vi "Amb_Factorial.vi"() -> ()   [LabVIEW 2015]
uses:
  <vilib>/Platform/TimedLoop/XDataNode/timing_clust.ctl
  <vilib>/Platform/TimedLoop/XDataNode/nitl_modes.ctl
  <vilib>/Platform/TimedLoop/XDataNode/wakeup.ctl
  <vilib>/DAQmx/read.llb/DAQmx Read (Analog DBL 1Chan 1Samp).vi
  <vilib>/DAQmx/read.llb/DAQmx Read (Analog 1D DBL NChan 1Samp).vi
  <vilib>/DAQmx/create/channels.llb/DAQmx Create Channel (AI-Voltage-Basic).vi
  <vilib>/Enthought/Python Integration Toolkit/api/Unpack Double.vi
  <vilib>/DAQmx/miscellaneous.llb/DAQmx Fill In Error Info.vi
  <vilib>/Platform/TimedLoop/XDataNode/XDataNode.xnode
  Program Files/neMESYS_SDK/neMESYS LabVIEW Kit/neMESYS LabVIEW Integration Kit.lvlib
  <vilib>/Platform/TimedLoop/XDataNode/XDNodeRunTimeDep.lvlib
  Conor/Temp CN7500/Omega CN7500/Omega CN7500.lvlib
  <vilib>/Enthought/Python Integration Toolkit/Python Integration Toolkit.lvlib
panel:
  out "Chi Sq 8":dbl
  out "Chi Sq ref 8":dbl
  out "Param 3 8":dbl
  out "Param 2 8":dbl
  out "Param 1 8":dbl
  out "Chi Sq 7":dbl
  out "Chi Sq ref 7":dbl
  out "Param 3 7":dbl
  out "Param 2 7":dbl
  out "Param 1 7":dbl
  out "Chi Sq 6":dbl
  out "Chi Sq ref 6":dbl
  out "Param 3 6":dbl
  out "Param 2 6":dbl
  out "Param 1 6":dbl
  out "Chi Sq 5":dbl
  out "Chi Sq ref 5":dbl
  out "Param 3 5":dbl
  out "Param 2 5":dbl
  out "Param 1 5":dbl
  out "Chi Sq 4":dbl
  out "Chi Sq ref 4":dbl
  out "Param 3 4":dbl
  out "Param 2 4":dbl
  out "Param 1 4":dbl
  in  "Cat Diameter um (eg 825)":dbl
  in  "Cat Mass G (EG 0.1)":dbl
  out "Exp 2":bool
  out "C EB 1":dbl
  out "C BAcid 1":dbl
  out "Exp 9":bool
  out "Liquid Inlet Pressure (bar g)":dbl
  in  "Liquid P sensor Terminal Configuration":i32(ring)=-1 items=["default"=-1, "RSE"=10083, "NRSE"=10078, "Differential"=10106, "Pseudodifferential"=12529]
  in  "Liquid P sensor Physical Channel":tag="Dev1/ai0"
  in  "Temp 2":dbl
  in  "Conc 2":dbl
  in  "Flow 2":dbl
  out "Exp 8":bool
  out "Exp 7":bool
  out "Exp 6":bool
  out "Exp 5":bool
  out "Exp 4":bool
  out "Exp 3":bool
  out "Exp 1":bool
  out "Exp 0":bool
  out "C BAcid 8":dbl
  out "C EB 8":dbl
  in  "Flow 8":dbl
  in  "Conc 8":dbl
  in  "Temp 8":dbl
  out "Temp 8":dbl
  out "Flow 8":dbl
  out "Conc 8":dbl
  out "C BAcid 7":dbl
  out "C EB 7":dbl
  in  "Flow 7":dbl
  in  "Conc 7":dbl
  in  "Temp 7":dbl
  out "Temp 7":dbl
  out "Flow 7":dbl
  out "Conc 7":dbl
  out "C BAcid 6":dbl
  out "C EB 6":dbl
  in  "Flow 6":dbl
  in  "Conc 6":dbl
  in  "Temp 6":dbl
  out "Temp 6":dbl
  out "Flow 6":dbl
  out "Conc 6":dbl
  out "C BAcid 5":dbl
  out "C EB 5":dbl
  in  "Flow 5":dbl
  in  "Conc 5":dbl
  in  "Temp 5":dbl
  out "Temp 5":dbl
  out "Flow 5":dbl
  out "Conc 5":dbl
  out "C BAcid 4":dbl
  out "C EB 4":dbl
  out "Conc 1":dbl
  out "Flow 1":dbl
  out "Temp 1":dbl
  out "Conc 2":dbl
  out "Flow 2":dbl
  out "Temp 2":dbl
  in  "Flow 4":dbl
  in  "Conc 4":dbl
  in  "Temp 4":dbl
  out "Temp 4":dbl
  out "Flow 4":dbl
  out "Conc 4":dbl
  out "C BAcid 3":dbl
  out "C EB 3":dbl
  out "Conc 3":dbl
  out "Flow 3":dbl
  out "Temp 3":dbl
  out "C BAcid 2":dbl
  out "C EB 2":dbl
  in  "Temp 3":dbl
  in  "Conc 3":dbl
  in  "Flow 3":dbl
  in  "Result file name -  needs extension .xlsx":string
  in  "HPLC file Name -doesnt need extension":string
  out "Desired Conc Not Possible":bool
  in  "Safety or Emergency Syringe Control":bool
  out "Feed Concentration (M)":dbl
  out "Total Flowrate (uL/min)":dbl
  out "Gas Back Pressure (barg)":dbl
  in  "Shut down in empty?\nLeft off, right on":bool
  in  "Clear":bool
  out "Safety Shut Down Pressure (barg)":dbl
  out "Calculated Pressure":dbl[](graph)
  out "Safety Shut Down Temp":dbl
  out "Actual Temp (oC)":dbl
  out "Temperature":dynamicdata(graph)
  out "Temp Set Point (oC)":dbl
  in  "Temp 1":dbl
  in  "Temp 0":dbl
  in  "Update Temperature Set Point":bool
  in  "Automated Experiments or Direct Control":bool
  in  "Set Point (oC)":dbl
  out "loop ind":dbl
  in  "Stop everything":bool
  in  "Skip Exp":bool
  in  "Minutes between Exp":dbl min=0.0 step=0.05
  in  "Refill 4":bool
  in  "Refill 3":bool
  in  "Refill 2":bool
  in  "Refill 1":bool
  in  "Empty 4":bool
  in  "Empty 3":bool
  in  "Empty 2":bool
  in  "Empty 1":bool
  in  "Calibrate 4":bool
  in  "Calibrate 3":bool
  in  "Calibrate 2":bool
  in  "Calibrate 1":bool
  in  "Stop Dose 4":bool
  in  "Stop Dose 3":bool
  in  "Stop Dose 2":bool
  in  "Stop Dose 1":bool
  in  "Flow 1":dbl
  in  "Conc 1":dbl
  in  "Flow 0":dbl
  in  "Conc 0":dbl
  in  "Generate Flow":bool
  in  "Set Flowrate 1":dbl
  in  "Set Flowrate 2":dbl
  in  "Set Flowrate 3":dbl
  in  "Set Flowrate 4":dbl
  in  "High Conc":dbl min=0.0 max=2.0
  in  "Low Conc":dbl min=0.0 max=2.0
  out "Syringe Level 4":dbl(slide) scale=0.0..5500.0
  out "Syringe Level 3":dbl(slide) scale=0.0..5500.0
  out "Syringe Level 2":dbl(slide) scale=0.0..5500.0
  out "Syringe Level 1":dbl(slide) scale=0.0..5500.0
  out "Flowrate 4 High":dbl
  out "Flowrate 3 High":dbl
  out "Flowrate 2 Low":dbl
  out "Flowrate 1 Low":dbl
  # "Pre Planned Experiments"
  # "Conducted Experiments Set Points"
  # "Current Conditions"
  # "1 & 2 chosen in advance"
  # "(uL/min)"
  # "3 onwards MBDoE"
  # "Coerced to nearest possible"
  # "Reported Values are set point no actual\nso if set point is not possible\ncoercion takes place\nbut actual is not recorded"
  # "Experimental Info"
  # "Factorial Only"
  # "example file name to show correct format is..."
  # "MBDoE2peakin1"
  # "Direct Control"
  # "Emergency Syringe Control Below"
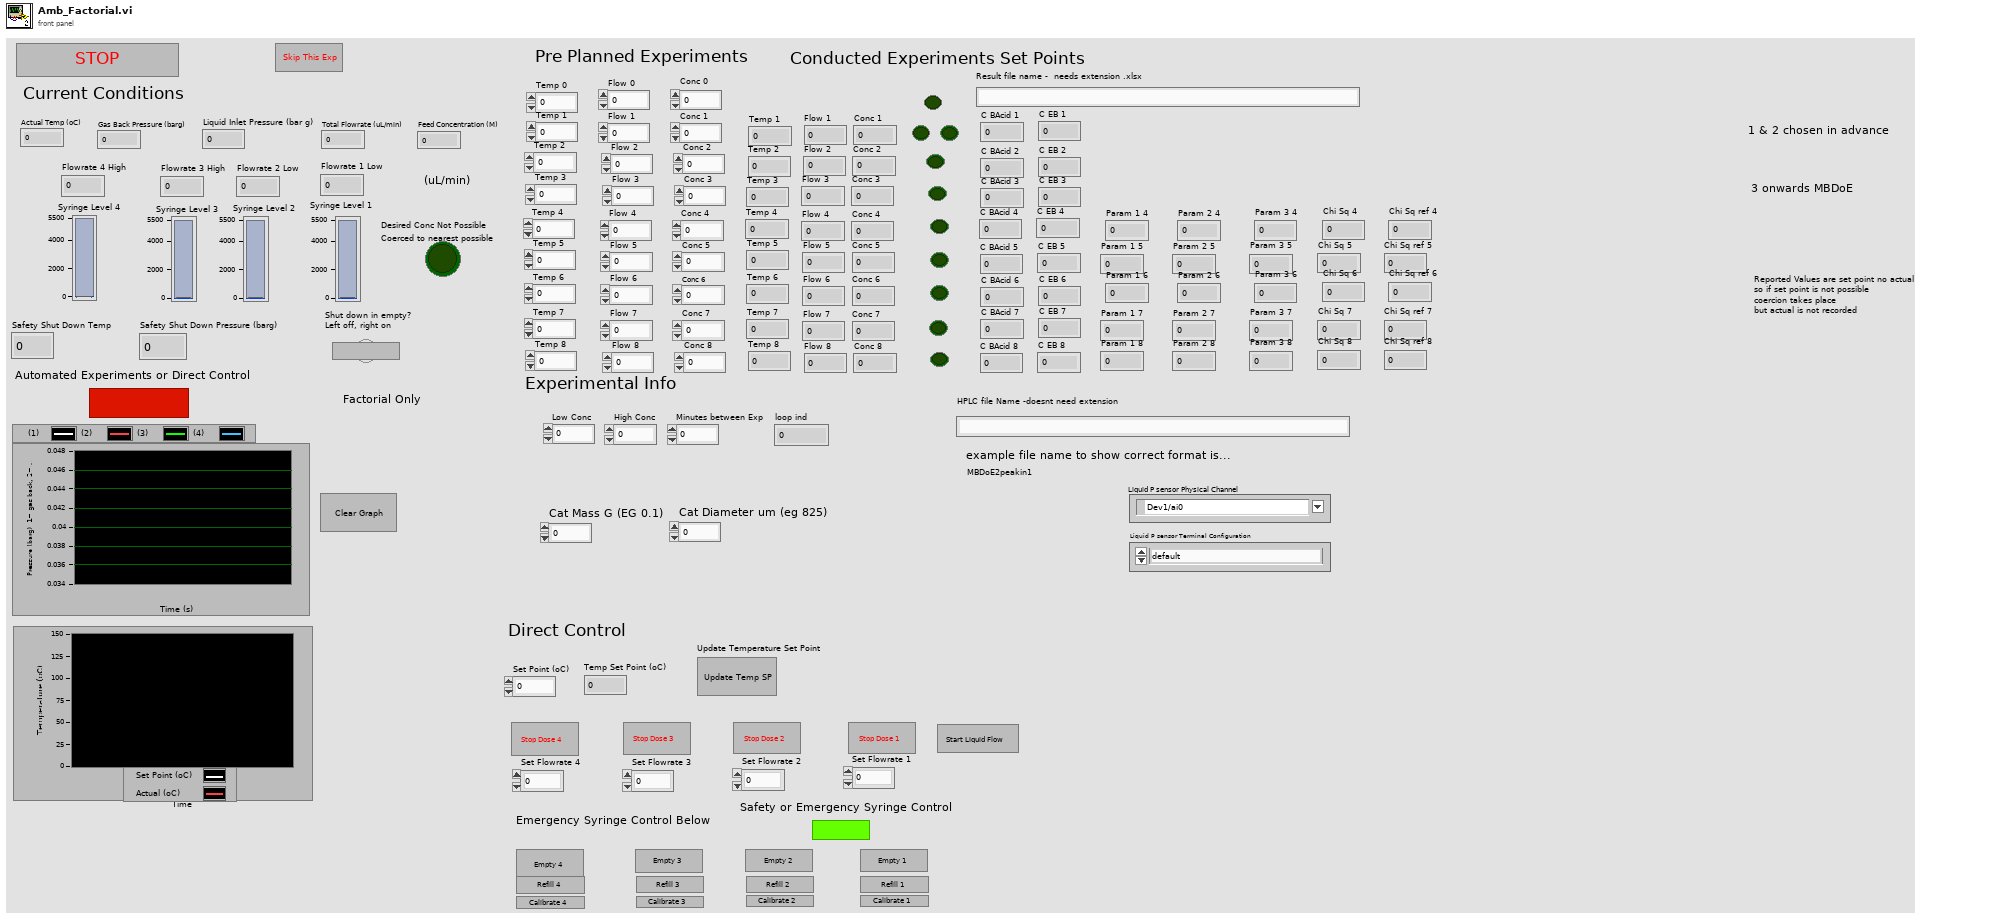
[diagram p1: front panel]
types:
  T1 = typedef "XDNodeRunTimeDep.lvlib/timing_clust.ctl" = cluster{"Expected End [f-1]":u64, "Actual End [f-1]":u64, "Finished Late? [f-1]":bool, "Expected End [i-1]":u64, "Actual End [i-1]":u64, "Finished Late? [i-1]":bool, "Expected Start [i]":u64, "Actual Start [i]":u64, "Expected Start [f]":u64, "Actual Start [f]":u64, "Source Name":string, "Structure Name":string, "Period":i64, "Deadline":i64, "Offset":i64, "Start":i64, "Priority":i32, "Timeout":i32, "Mode":T2, "Wakeup Reason":T3, "Error":errorcluster, "Source Type":string, "Secondary Source Type":string, "Global End Time":u64, "Global Start Time":u64, "Frame Duration":u64, "Iteration Duration":u64, "Assigned CPU":i32, "I/O Scan Engine Mode":u32}
  T2 = typedef "XDNodeRunTimeDep.lvlib/nitl_modes.ctl" = enum32{"No Change", "Process missed periods, maintain original phase", "Discard missed periods, maintain original phase", "Process missed periods, ignore original phase", "Discard missed periods, ignore original phase"}
  T3 = typedef "XDNodeRunTimeDep.lvlib/wakeup.ctl" = enum32{"Normal", "Aborted", "Asynchronous wakeup", "Timing source error", "Timed loop error", "Timeout"}
  T4 = typedef "Python Integration Toolkit.lvlib/Session ID.ctl" = u64
  T5 = typedef "Python Integration Toolkit.lvlib/Python Objects.ctl" = variant
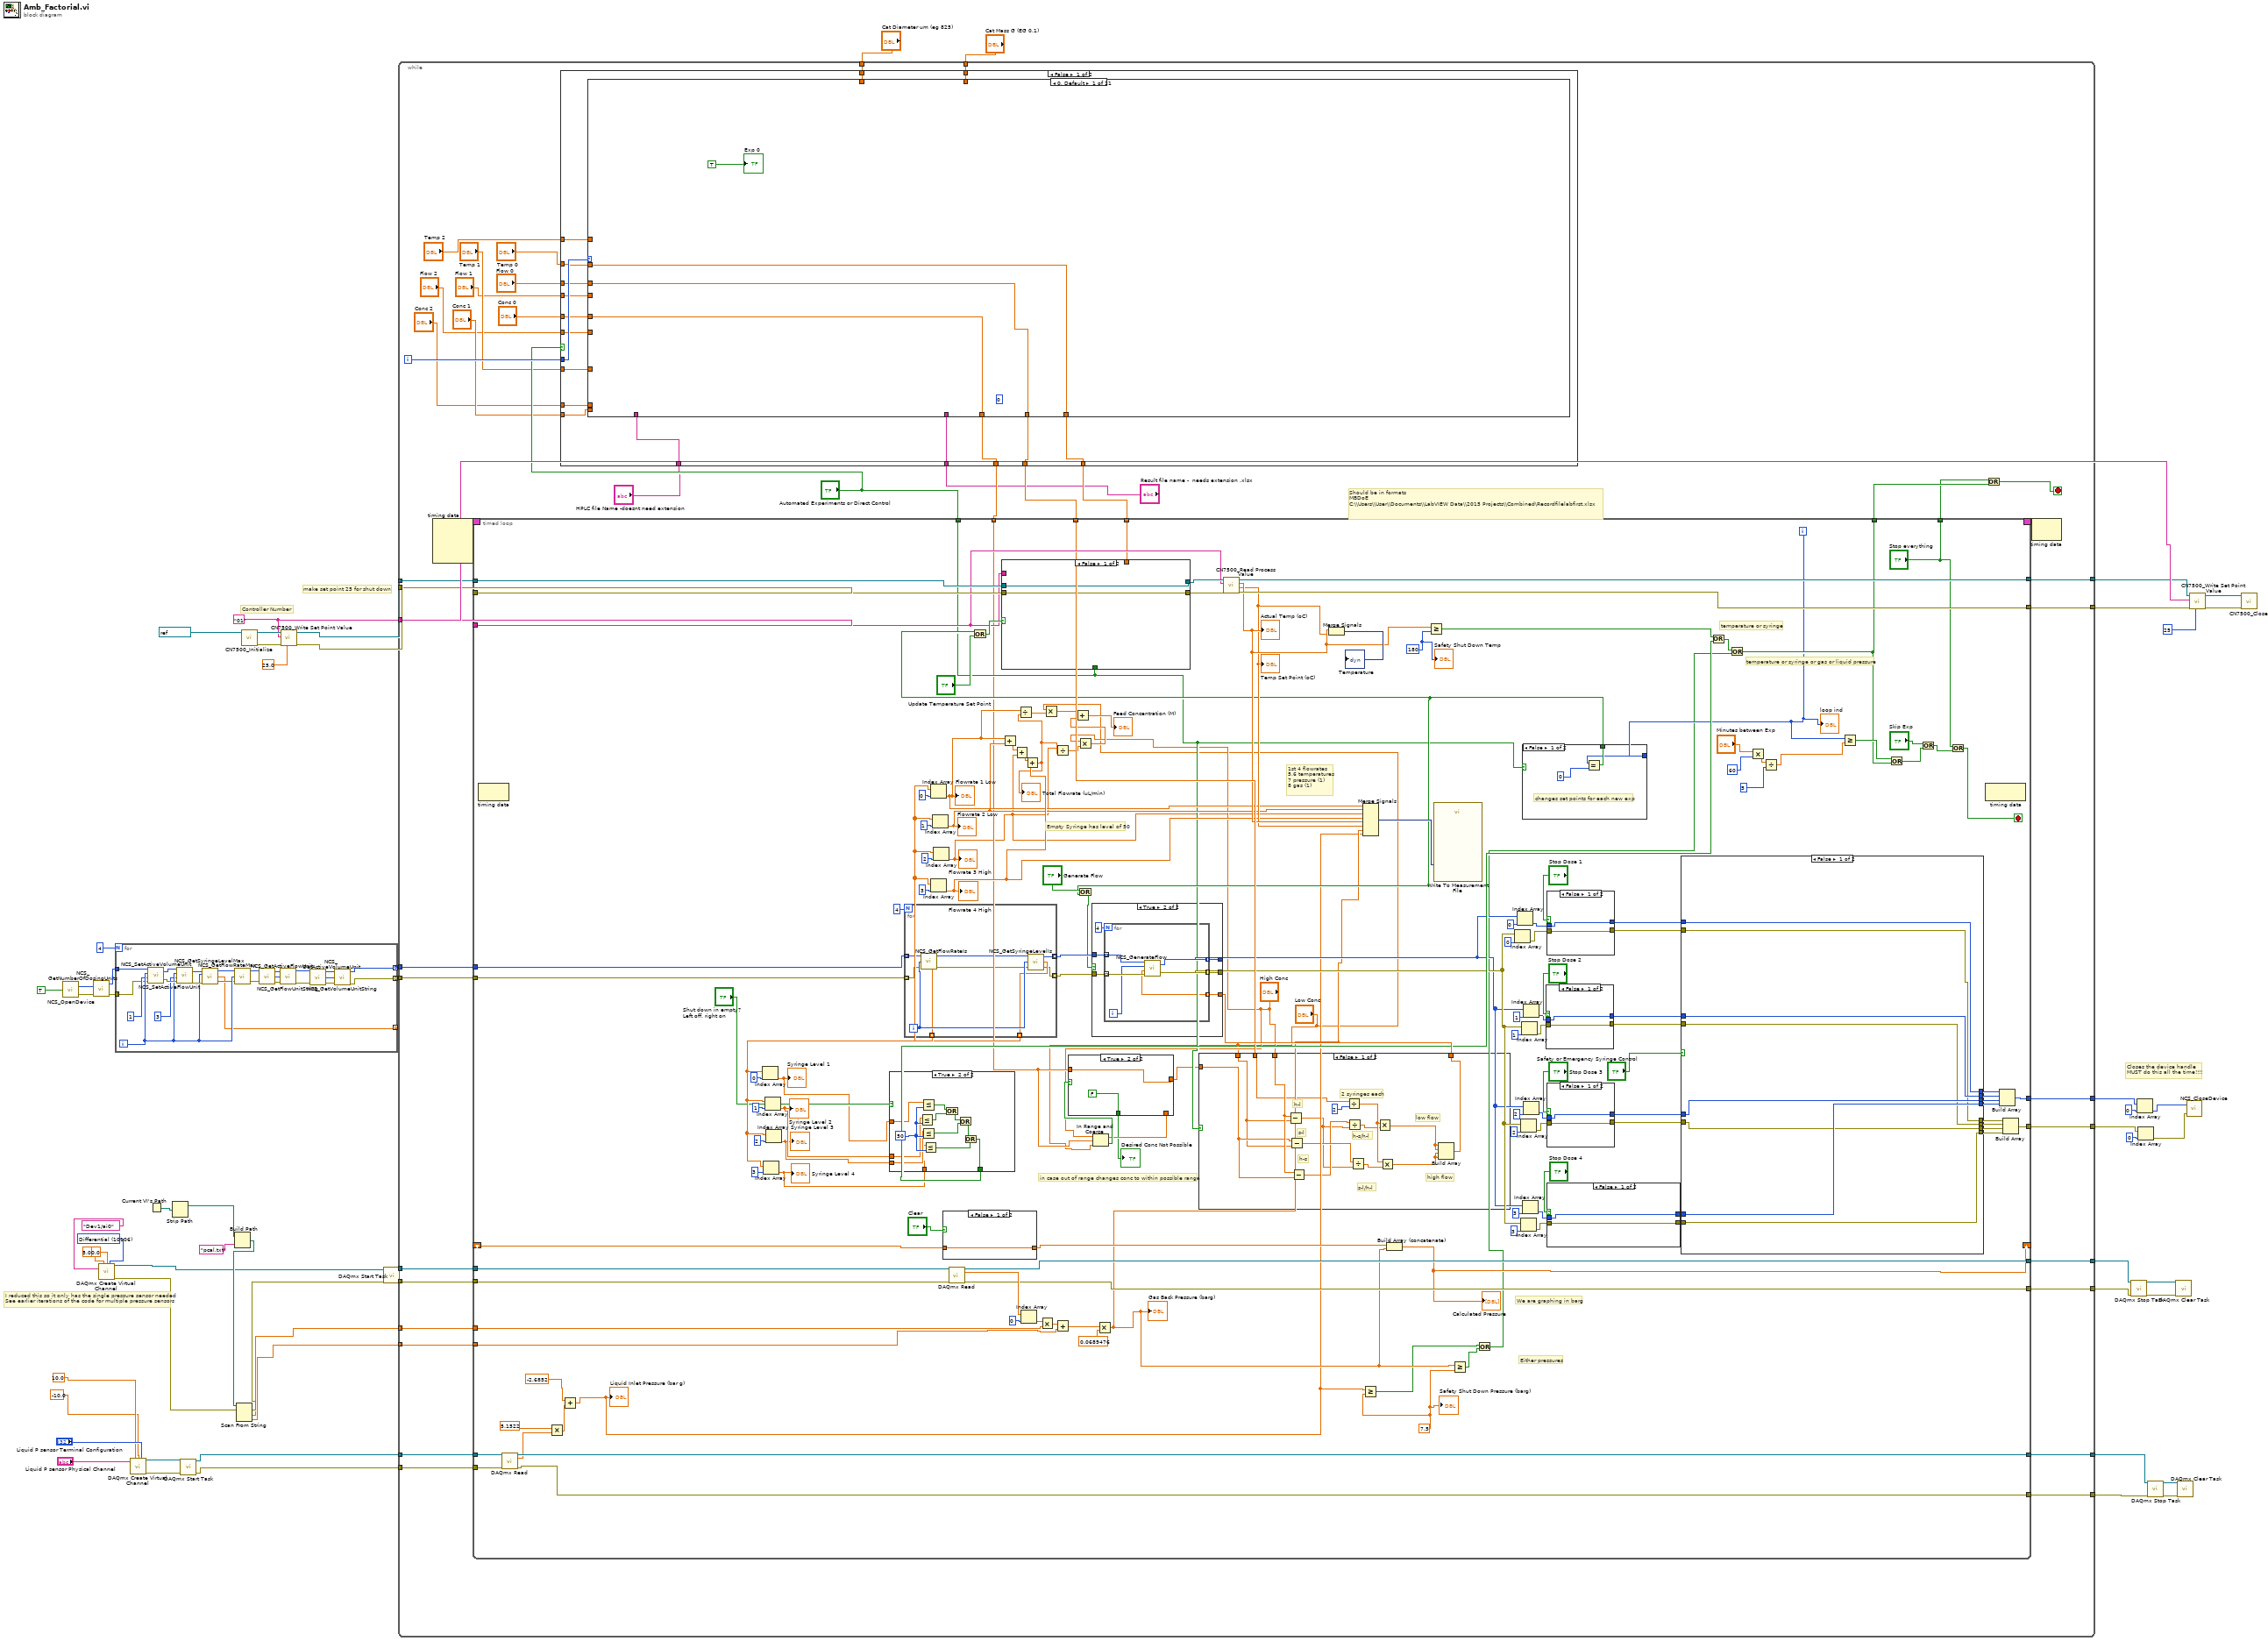
[diagram p0: block diagram]
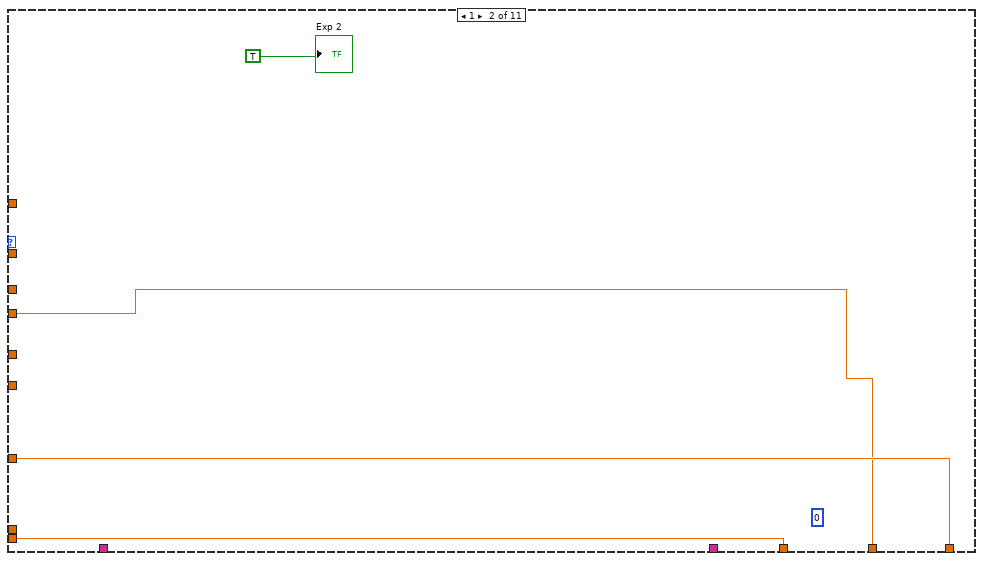
[diagram p2: hidden frame]
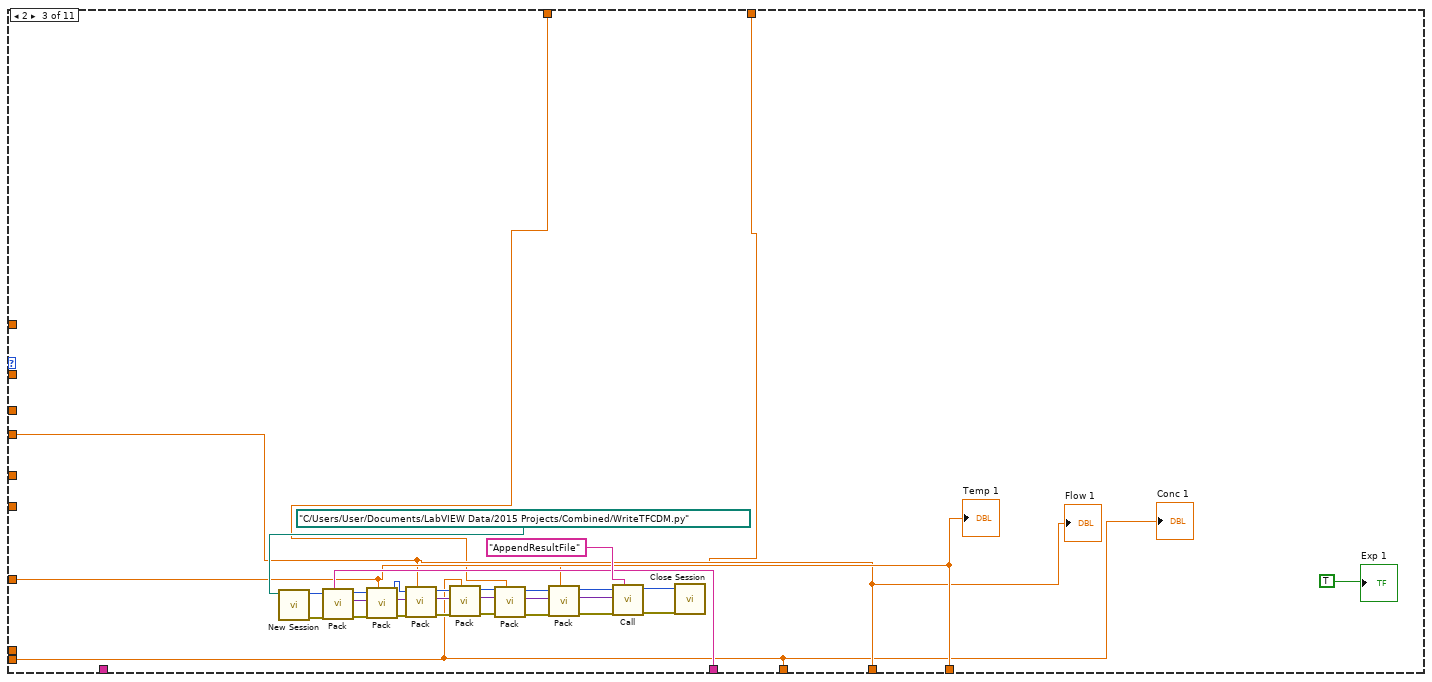
[diagram p3: hidden frame]
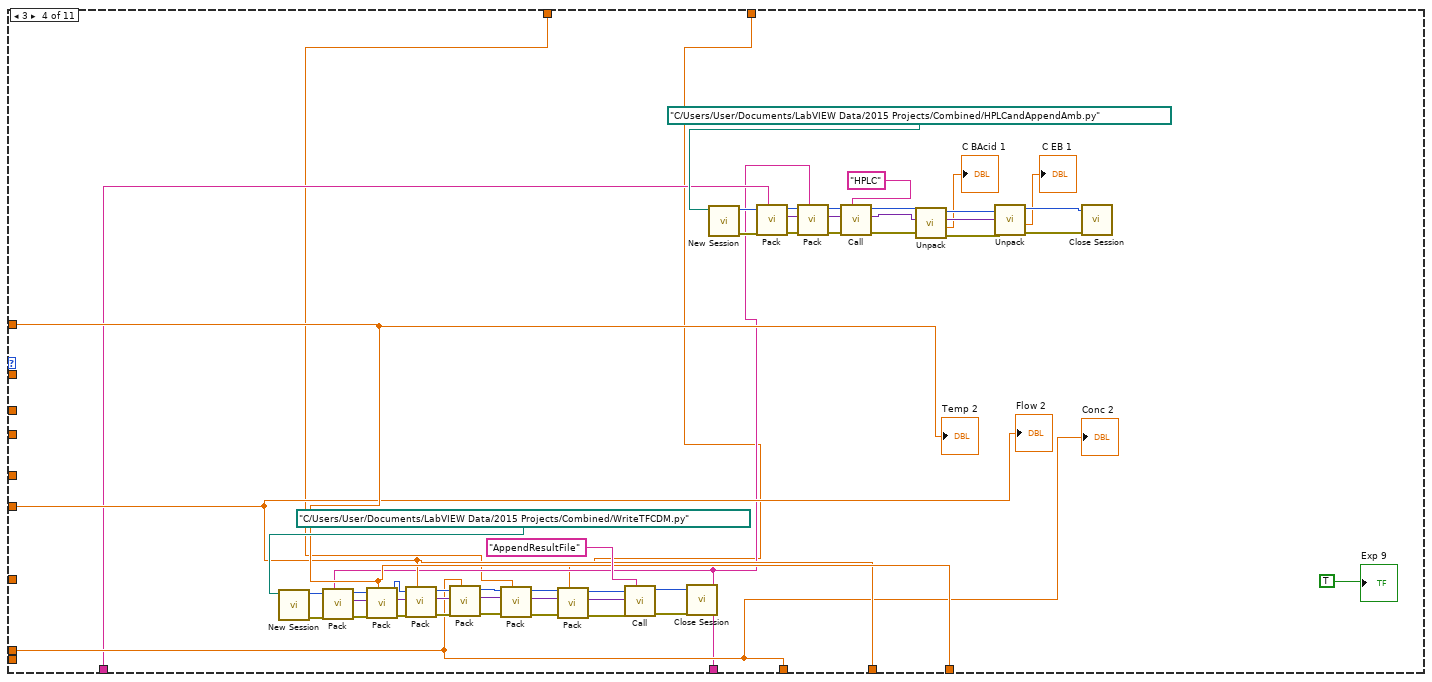
[diagram p4: hidden frame]
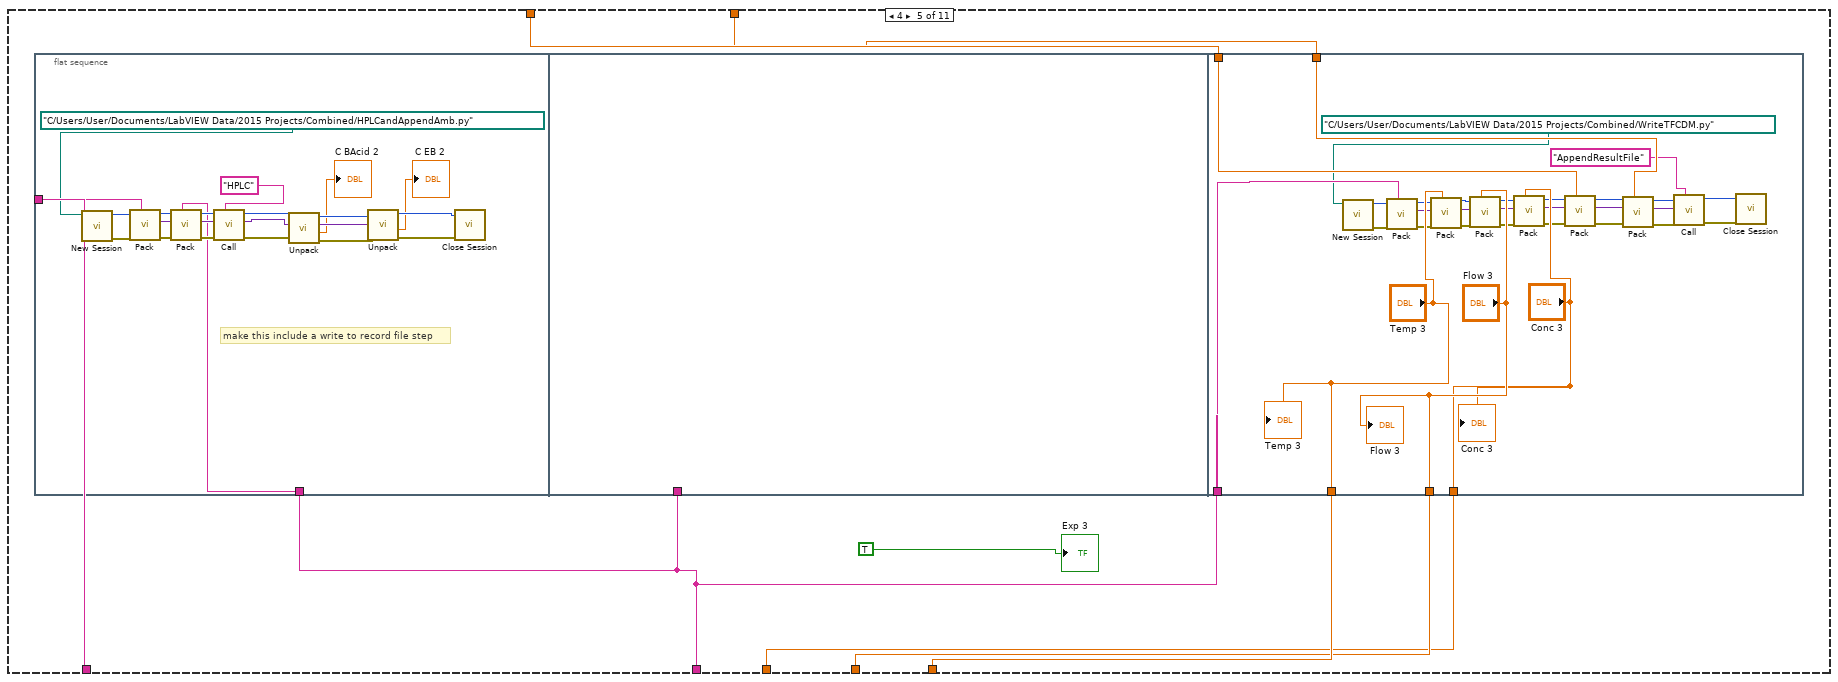
[diagram p5: hidden frame]
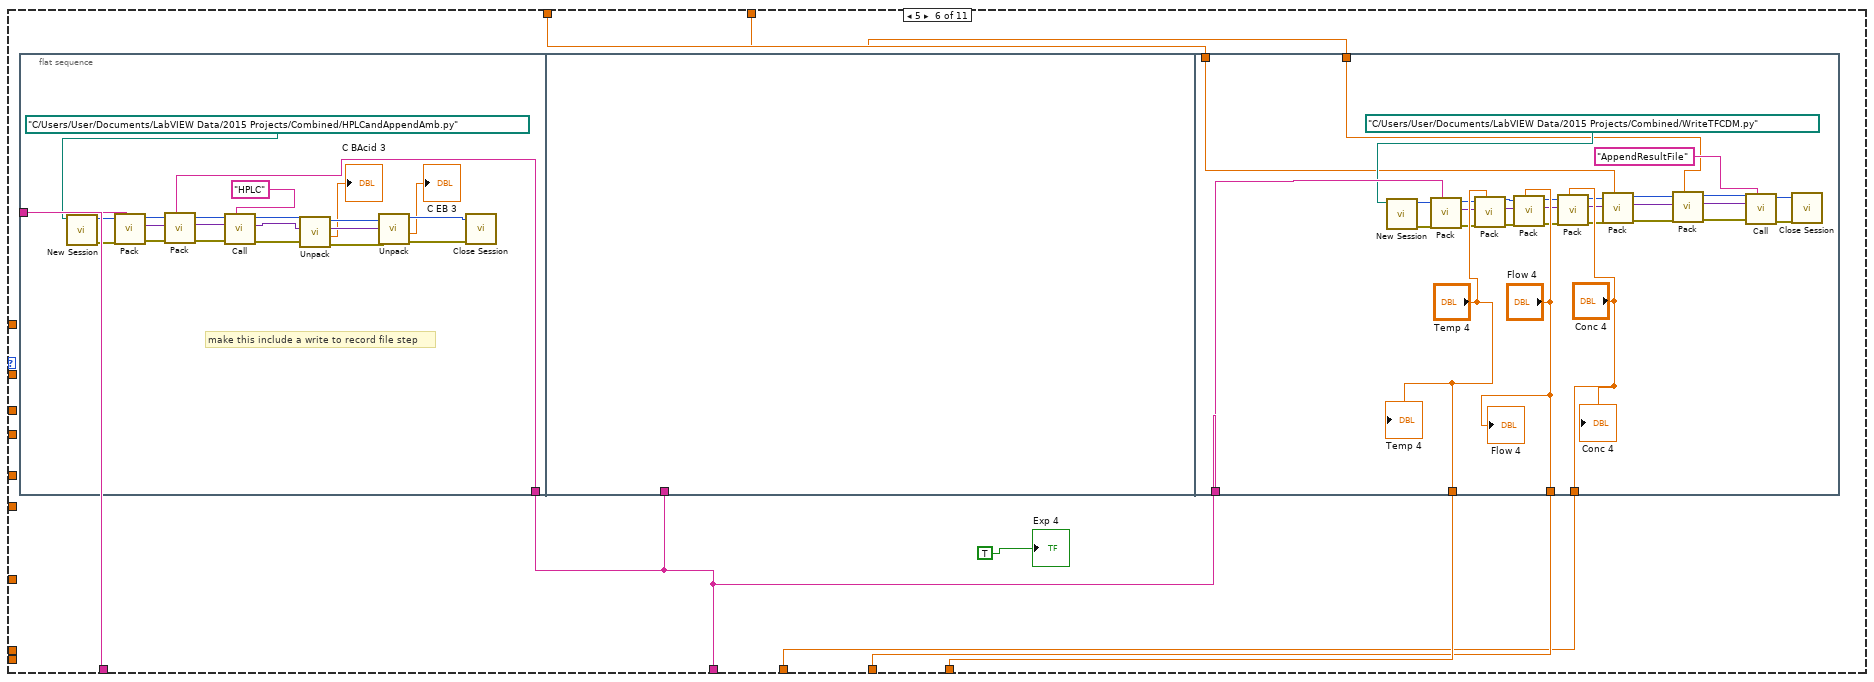
[diagram p6: hidden frame]
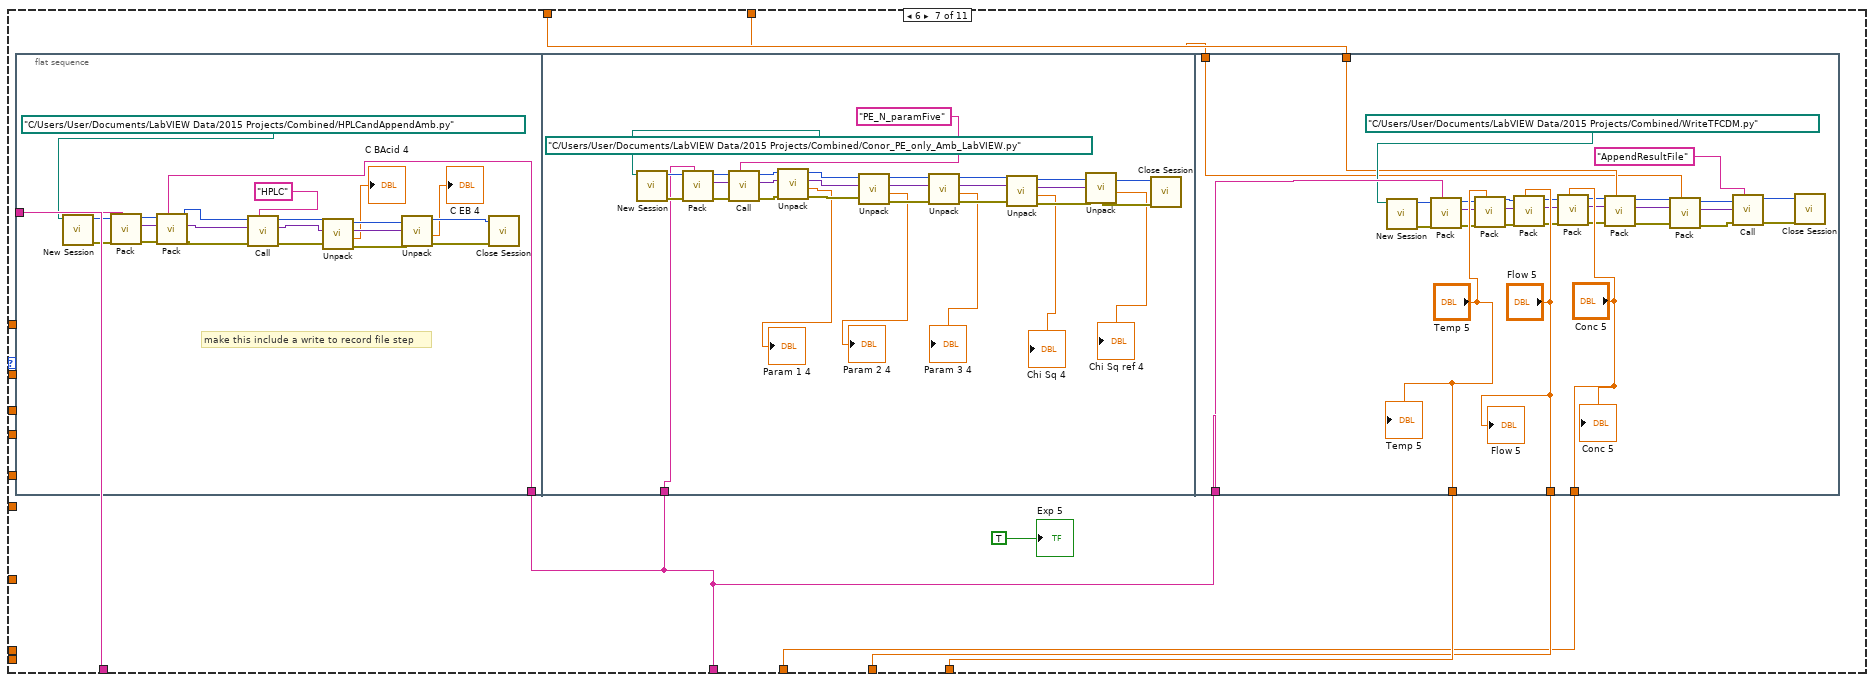
[diagram p7: hidden frame]
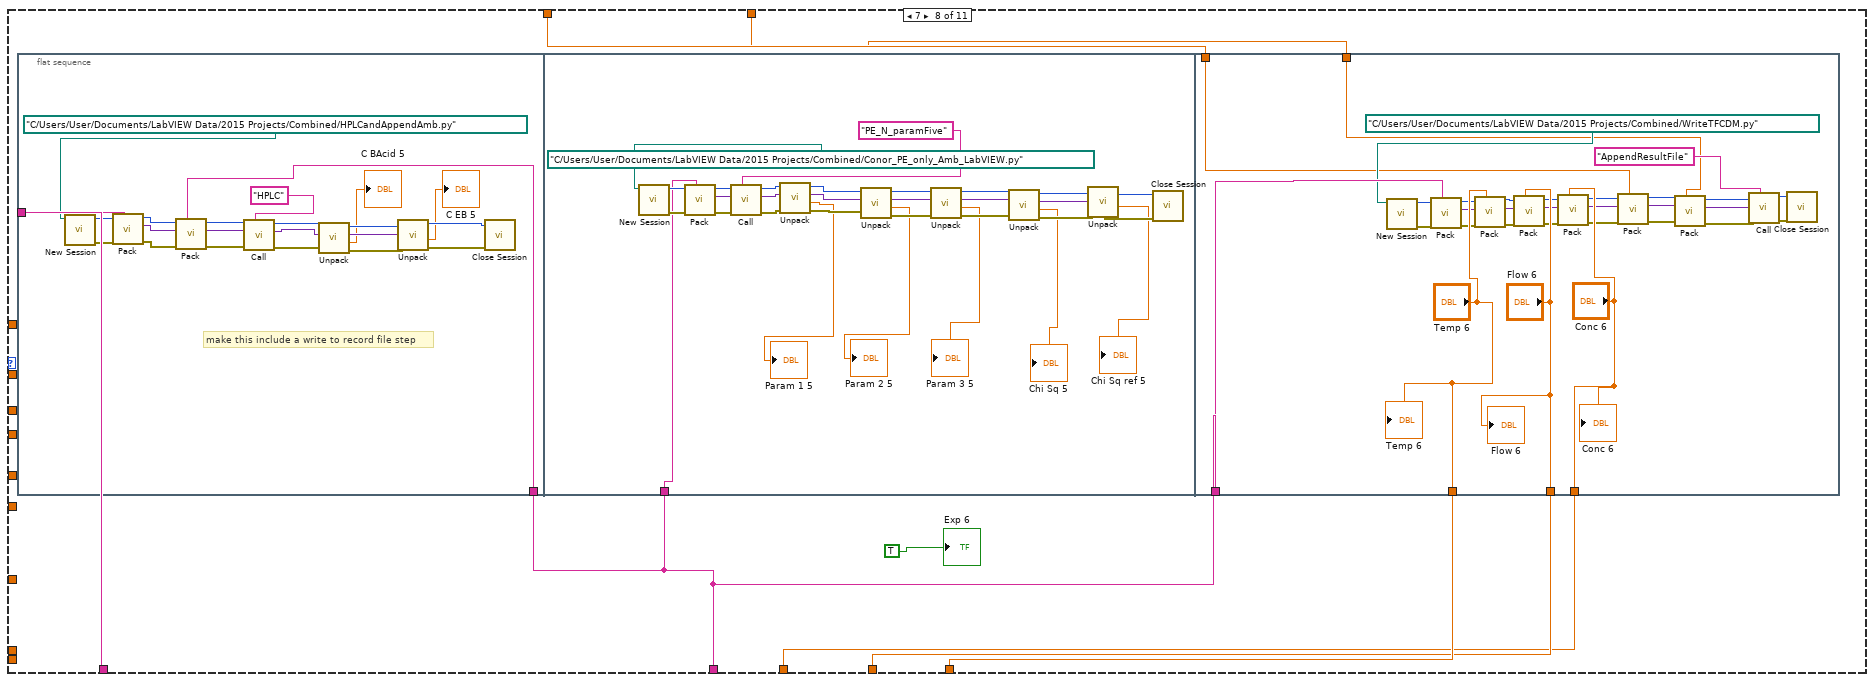
[diagram p8: hidden frame]
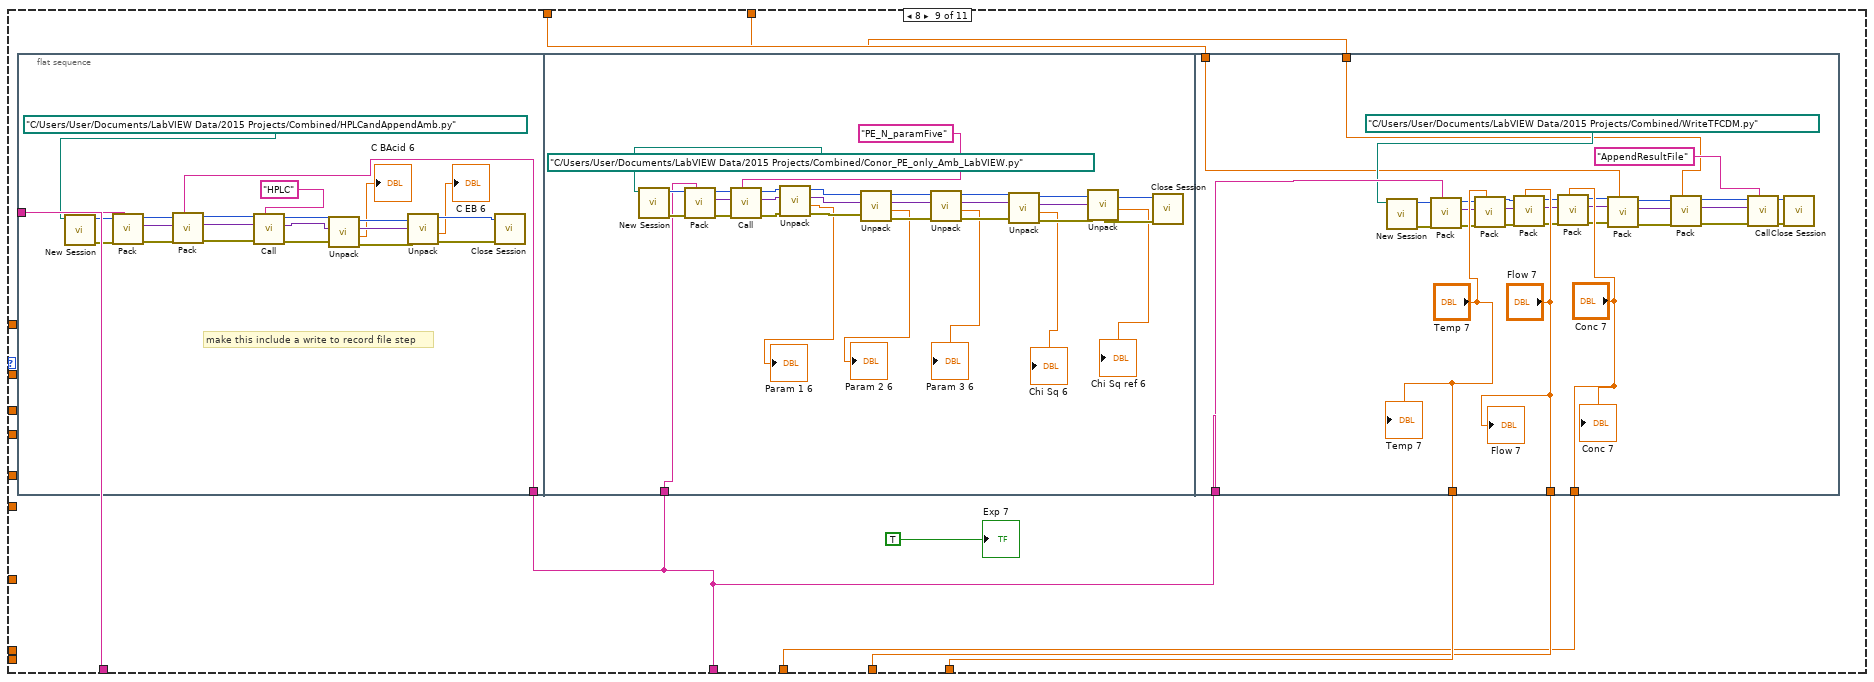
[diagram p9: hidden frame]
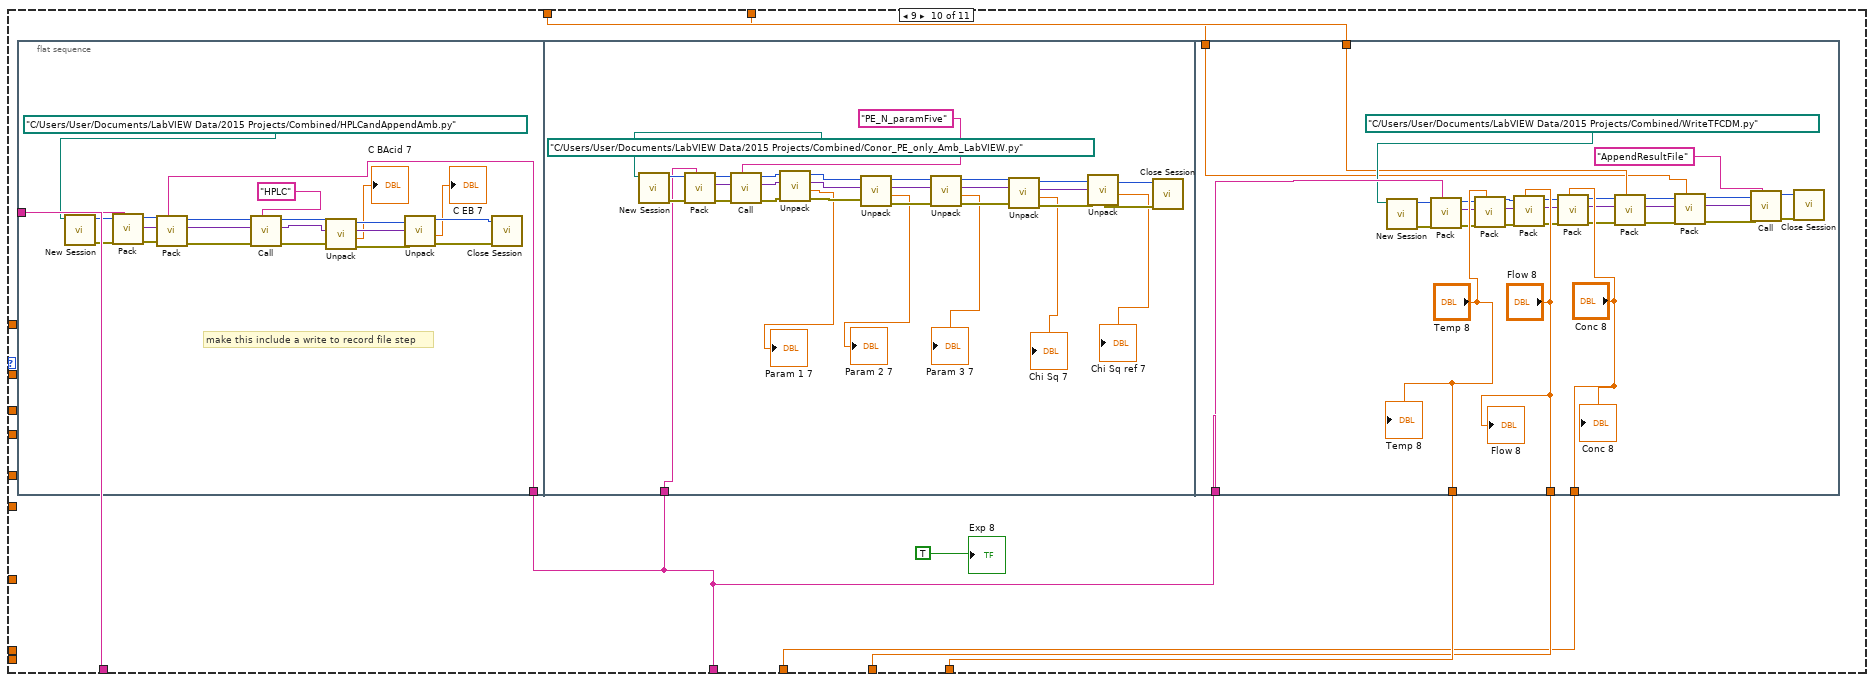
[diagram p10: hidden frame]
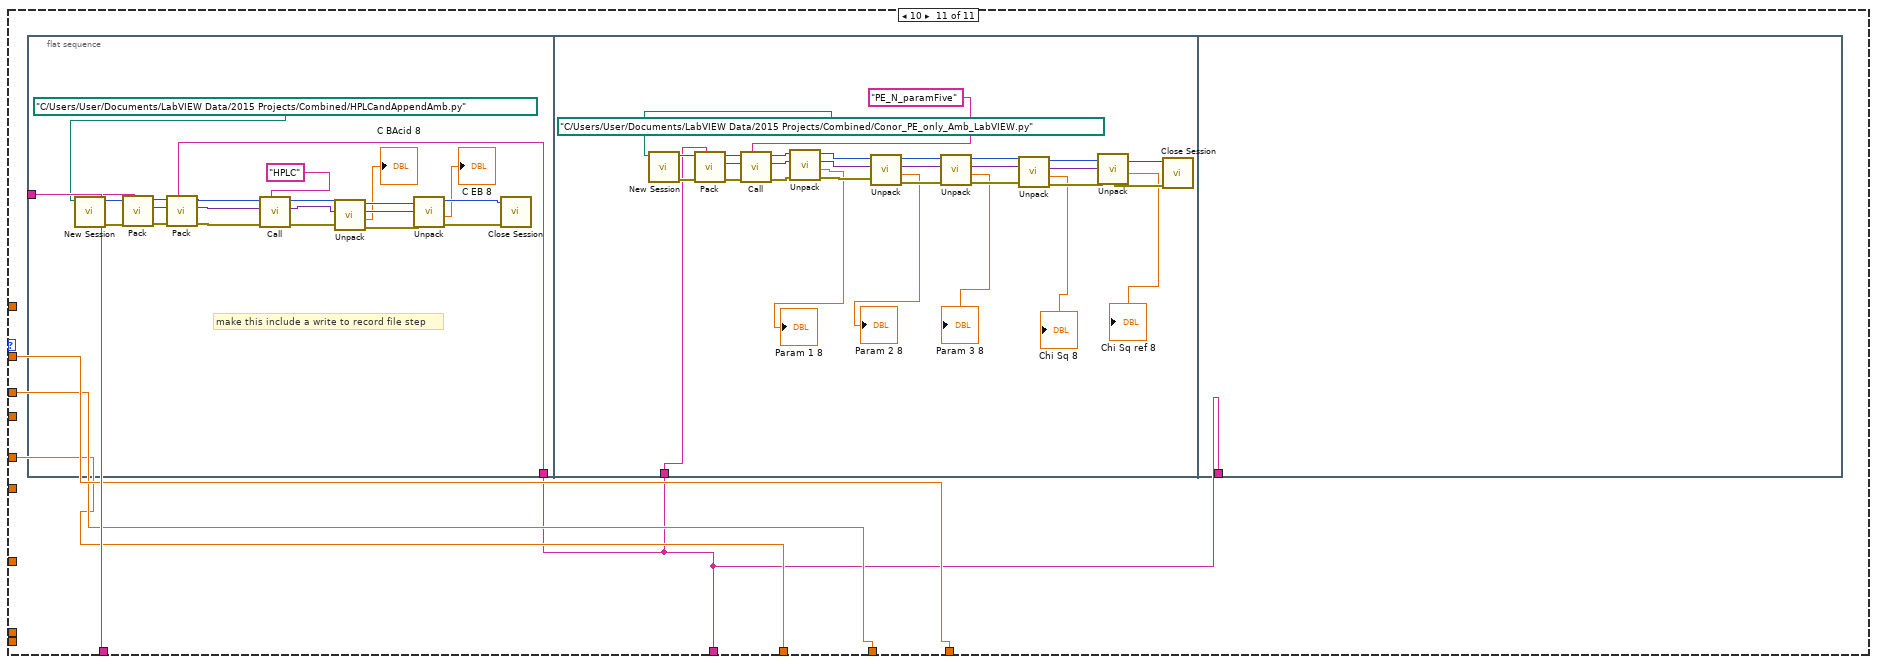
[diagram p11: hidden frame]
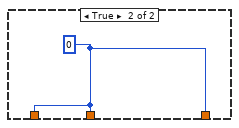
[diagram p12: hidden frame]
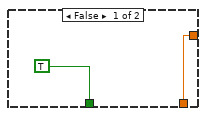
[diagram p13: hidden frame]
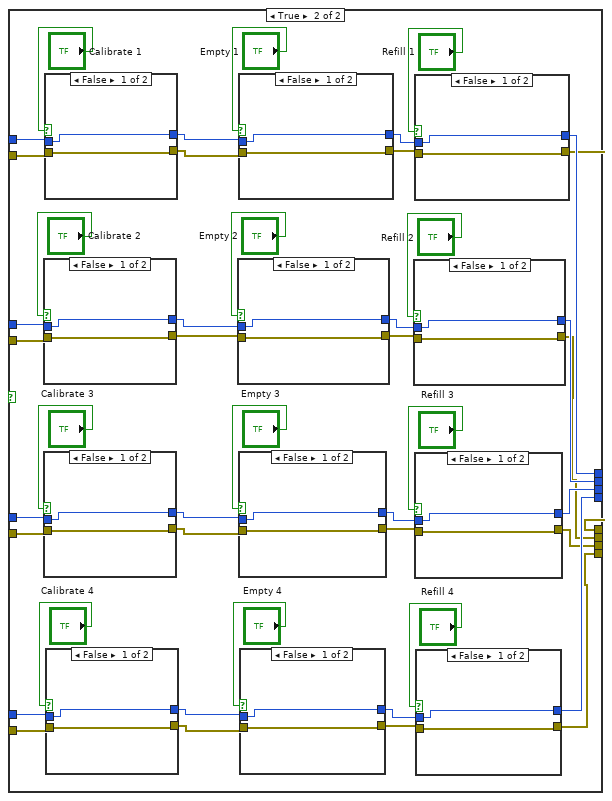
[diagram p14: hidden frame]
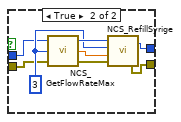
[diagram p15: hidden frame]
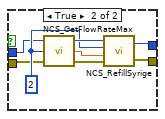
[diagram p16: hidden frame]
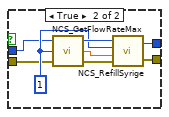
[diagram p17: hidden frame]
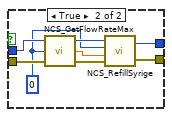
[diagram p18: hidden frame]
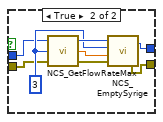
[diagram p19: hidden frame]
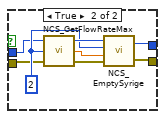
[diagram p20: hidden frame]
diagram:
  w31 = 10106 items=["default"=-1, "RSE"=10083, "NRSE"=10078, "Differential"=10106, "Pseudodifferential"=12529] ("input terminal configuration")
  w38 = "01" ("Controller Number")
  # "I reduced this so it only has the single pressure sensor needed\nSee earlier iterations of the code for multiple pressure sensors"
  # "make set point 25 for shut down"
  # "Controller Number"
  # "Closes the device handle \nMUST do this all the time!!!!"
  n1 = call "NCS_OpenDevice.vi"("show status window"=TRUE) -> ("device handle"=w57:u32, "error out"=w56:errorcluster)
  n2 = call "NCS_GetNumberOfDosingUnits.vi"("device handle in"=w57, "error in (no error)"=w56) -> ("device handle out"=w54:u32, "error out"=w55:errorcluster)  [unwired: 1 out]
  n3 = call-poly <vilib>:"DAQmx Create Virtual Channel.vi"("maximum value"=5.0, "minimum value"=0.0, "input terminal configuration"=w31, "physical channels"=tag "Dev1/ai0") -> ("task out"=w15:refnum<k21>, "error out"=w16:errorcluster)  [unwired: 10 in]
  n4 = for {
    N: 4 -> [_]
    tunnel: [w63] -> w53 mode=indexing
    tunnel: [w62] -> w52 mode=indexing
    tunnel: [w76] -> _ mode=indexing
    tunnel: w55 -> [w61]
    tunnel: w54 -> [w60]
    i -> [w79]
    n5 = call "NCS_SetActiveVolumeUnit.vi"("error in (no error)"=w61, "active volume unit"=1, "dosingunit"=w79, "device handle in"=w60) -> ("error out"=w82:errorcluster, "device handle out"=w83:u32)
    n6 = call "NCS_SetActiveFlowUnit.vi"("error in (no error)"=w82, "active flow unit"=3, "dosingunit"=w79, "device handle in"=w83) -> ("error out"=w80:errorcluster, "device handle out"=w81:u32)
    n7 = call "NCS_GetSyringeLevelMax.vi"("error in (no error)"=w80, "dosingunit"=w79, "device handle in"=w81) -> ("error out"=w77:errorcluster, "syringe level max"=w76:dbl, "device handle out"=w78:u32)  [unwired: 1 out]
    n8 = call "NCS_GetFlowRateMax.vi"("error in (no error)"=w77, "dosingunit"=w79, "device handle in"=w78) -> ("error out"=w64:errorcluster, "device handle out"=w65:u32)  [unwired: 1 out]
    n9 = call "NCS_GetActiveFlowUnit.vi"("error in (no error)"=w64, "device handle in"=w65) -> ("error out"=w72:errorcluster, "active flow unit"=w71:u8, "device handle out"=w73:u32)  [unwired: 1 in]
    n10 = call "NCS_GetFlowUnitString.vi"("device handle in"=w73, "flow unit id"=w71, "error in (no error)"=w72) -> ("device handle out"=w68:u32, "error out"=w67:errorcluster)  [unwired: 2 out]
    n11 = call "NCS_GetActiveVolumeUnit.vi"("error in (no error)"=w67, "device handle in"=w68) -> ("error out"=w69:errorcluster, "active volume unit"=w70:u8, "device handle out"=w66:u32)  [unwired: 1 in]
    n12 = call "NCS_GetVolumeUnitString.vi"("device handle in"=w66, "volume unit id"=w70, "error in (no error)"=w69) -> ("device handle out"=w63:u32, "error out"=w62:errorcluster)  [unwired: 2 out]
  }
  n13 = call-poly <vilib>:"DAQmx Create Virtual Channel.vi"("maximum value"=10.0, "minimum value"=-10.0 ("maximum value"), "input terminal configuration"="Liquid P sensor Terminal Configuration", "physical channels"="Liquid P sensor Physical Channel") -> ("task out"=w11:refnum<k21>, "error out"=w12:errorcluster)  [unwired: 10 in]
  n14 = Current VI's Path() -> (path=w29:path)
  n15 = Strip Path(path=w29) -> (stripped path=w27:path)  [unwired: 1 out]
  n16 = call <vilib>:"DAQmx Start Task.vi"("task/channels in"=w11, "error in"=w12) -> ("task out"=w10:refnum<k21>, "error out"=w9:errorcluster)  [unwired: 12 in]
  n17 = Build Path(base path=w27, name or relative path="pcal.txt") -> (appended path=w28:path)
  n18 = Scan From String(w28, w16) -> (w25:errorcluster, output 1=w22:dbl, output 2=w21:dbl)  [unwired: 3 in, 1 out]
  n19 = call "CN7500_Initialize.vi"("VISA resource name"=refnum<visa-resource-name> "COM8") -> ("error out"=w44:errorcluster, "VISA resource name out"=w45:refnum<visa-resource-name>)  [unwired: 9 in]
  n20 = call "CN7500_Write Set Point Value.vi"("Target Set Point Value"=25.0, "error in (no error)"=w44, "Controller Number"=w38, "VISA In"=w45) -> ("error out"=w36:errorcluster, "VISA Out"=w37:refnum<visa-resource-name>)  [unwired: 6 in]
  n21 = call <vilib>:"DAQmx Start Task.vi"("task/channels in"=w15, "error in"=w25) -> ("task out"=w24:refnum<k21>, "error out"=w23:errorcluster)  [unwired: 12 in]
  n22 = while {
    tunnel: w53 -> [w125]
    tunnel: w52 -> [w124]
    tunnel: [w123] -> w47
    tunnel: [w122] -> w46
    tunnel: w38 -> [w119]
    tunnel: w37 -> [w118]
    tunnel: w36 -> [w117]
    tunnel: [w116] -> w35
    tunnel: [w115] -> w34
    tunnel: w24 -> [w113]
    tunnel: w23 -> [w112]
    tunnel: w22 -> [w111]
    tunnel: w21 -> [w110]
    tunnel: [w109] -> w18
    tunnel: [w108] -> w17
    tunnel: w10 -> [w92]
    tunnel: w9 -> [w91]
    tunnel: [w90] -> w7
    tunnel: [w89] -> w5
    tunnel: "Cat Diameter um (eg 825)" -> [w85]
    tunnel: "Cat Mass G (EG 0.1)" -> [w84]
    i -> [w102]
    stop <- w107 stop-if-true
    # "Should be in formats \nMBDoE\nC:\\\\Users\\\\User\\\\Documents\\\\LabVIEW Data\\\\2015 Projects\\\\Combined\\Recordfilelabfirst.xlsx"
    n23 = node-c288() -> (w121:T1)  [unwired: 4 in]
    n24 = case shown="False" "Automated Experiments or Direct Control" {
      tunnel: [w139 w771] -> w105
      tunnel: [w137 w771] -> w104
      tunnel: [w141 w771] -> w103
      tunnel: w102 -> [w142 _]
      tunnel: "Conc 0" -> [w140 _]
      tunnel: "Flow 0" -> [w136 _]
      tunnel: "Temp 0" -> [w138 _]
      tunnel: "Temp 1" -> [w134 _]
      tunnel: "Flow 1" -> [w133 _]
      tunnel: "Conc 1" -> [w132 _]
      tunnel: "HPLC file Name -doesnt need extension" -> [w131 _]
      tunnel: "Result file name -  needs extension .xlsx" -> [w135 _]
      tunnel: "Temp 2" -> [w130 _]
      tunnel: "Flow 2" -> [w129 _]
      tunnel: "Conc 2" -> [w128 _]
      tunnel: w85 -> [w127 _]
      tunnel: w84 -> [w126 _]
      frame False {
        n25 = case shown="0, Default" w142 {
          tunnel: [w144 w147 w163 w215 w238 w298 w358 w448 w538 w628 w715] -> w141
          tunnel: w140 -> [w144 _ _ _ _ _ _ _ _ _ w715]
          tunnel: [w146 w149 w165 w217 w240 w300 w360 w450 w540 w630 w717] -> w139
          tunnel: w138 -> [w146 _ _ _ _ _ _ _ _ _ w717]
          tunnel: [w145 w148 w164 w216 w239 w299 w359 w449 w539 w629 w716] -> w137
          tunnel: w136 -> [w145 _ _ _ _ _ _ _ _ _ w716]
          tunnel: w135 -> [_ _ w166 w193 w237 w297 w357 w447 w537 w627 w714]
          tunnel: w134 -> [_ w149 w165 _ _ _ _ _ _ _ _]
          tunnel: w133 -> [_ w148 w164 _ _ _ _ _ _ _ _]
          tunnel: w132 -> [_ w147 w163 _ _ _ _ _ _ _ _]
          tunnel: w131 -> [_ _ _ w194 w241 w301 w361 w451 w541 w631 w718]
          tunnel: w130 -> [_ _ _ w217 _ _ _ _ _ _ _]
          tunnel: w129 -> [_ _ _ w216 _ _ _ _ _ _ _]
          tunnel: w128 -> [_ _ _ w215 _ _ _ _ _ _ _]
          tunnel: w127 -> [_ _ w161 w183 w235 w295 w355 w445 w535 w625 _]
          tunnel: w126 -> [_ _ w160 w182 w234 w294 w354 w444 w534 w624 _]
          frame 0, Default {
            (unwired) 0
            "Exp 0" <- TRUE
          }
          frame 1 {
            (unwired) 0
            "Exp 2" <- TRUE
          }
          frame 2 {
            n26 = call <vilib>:"New Session.vi"("Path to Python Module (.py File)"=path "C:/Users/User/Documents/LabVIEW Data/2015 Projects/Combined/WriteTFCDM.py") -> ("error out"=w173:errorcluster, "Session ID out"=w172:T4)  [unwired: 9 in]
            n27 = call <vilib>:"Pack.vi"("Argument"=w166, "error in (no error)"=w173, "Session ID"=w172) -> ("error out"=w174:errorcluster, "Python Object References Out"=w178:T5, "Session ID out"=w171:T4)  [unwired: 6 in]
            n28 = call <vilib>:"Pack.vi"("Argument"=w165, "error in (no error)"=w174, "Python Object References In"=w178, "Session ID"=w171) -> ("error out"=w175:errorcluster, "Python Object References Out"=w179:T5, "Session ID out"=w181:T4)  [unwired: 5 in]
            n29 = call <vilib>:"Pack.vi"("Argument"=w164, "error in (no error)"=w175, "Python Object References In"=w179, "Session ID"=w181) -> ("error out"=w176:errorcluster, "Python Object References Out"=w180:T5, "Session ID out"=w167:T4)  [unwired: 5 in]
            n30 = call <vilib>:"Pack.vi"("Argument"=w163, "error in (no error)"=w176, "Python Object References In"=w180, "Session ID"=w167) -> ("error out"=w153:errorcluster, "Python Object References Out"=w156:T5, "Session ID out"=w159:T4)  [unwired: 5 in]
            n31 = call <vilib>:"Pack.vi"("Argument"=w161, "error in (no error)"=w153, "Python Object References In"=w156, "Session ID"=w159) -> ("error out"=w152:errorcluster, "Python Object References Out"=w155:T5, "Session ID out"=w158:T4)  [unwired: 5 in]
            n32 = call <vilib>:"Pack.vi"("Argument"=w160, "error in (no error)"=w152, "Python Object References In"=w155, "Session ID"=w158) -> ("error out"=w151:errorcluster, "Python Object References Out"=w154:T5, "Session ID out"=w157:T4)  [unwired: 5 in]
            n33 = call <vilib>:"Call.vi"("Function or Method Name"="AppendResultFile", "error in (no error)"=w151, "Python Object References In"=w154, "Session ID"=w157) -> ("error out"=w177:errorcluster, "Session ID out"=w168:T4)  [unwired: 5 in, 1 out]
            n34 = call <vilib>:"Close Session.vi"("error in (no error)"=w177, "Session ID"=w168) -> ()  [unwired: 9 in, 1 out]
            "Temp 1" <- w165
            "Flow 1" <- w164
            "Conc 1" <- w163
            "Exp 1" <- TRUE
          }
          frame 3 {
            n35 = call <vilib>:"New Session.vi"("Path to Python Module (.py File)"=path "C:/Users/User/Documents/LabVIEW Data/2015 Projects/Combined/WriteTFCDM.py") -> ("error out"=w225:errorcluster, "Session ID out"=w224:T4)  [unwired: 9 in]
            n36 = call <vilib>:"Pack.vi"("Argument"=w193, "error in (no error)"=w225, "Session ID"=w224) -> ("error out"=w226:errorcluster, "Python Object References Out"=w230:T5, "Session ID out"=w223:T4)  [unwired: 6 in]
            n37 = call <vilib>:"Pack.vi"("Argument"=w217, "error in (no error)"=w226, "Python Object References In"=w230, "Session ID"=w223) -> ("error out"=w227:errorcluster, "Python Object References Out"=w231:T5, "Session ID out"=w233:T4)  [unwired: 5 in]
            n38 = call <vilib>:"Pack.vi"("Argument"=w216, "error in (no error)"=w227, "Python Object References In"=w231, "Session ID"=w233) -> ("error out"=w228:errorcluster, "Python Object References Out"=w232:T5, "Session ID out"=w219:T4)  [unwired: 5 in]
            n39 = call <vilib>:"Pack.vi"("Argument"=w215, "error in (no error)"=w228, "Python Object References In"=w232, "Session ID"=w219) -> ("error out"=w186:errorcluster, "Python Object References Out"=w189:T5, "Session ID out"=w192:T4)  [unwired: 5 in]
            n40 = call <vilib>:"Pack.vi"("Argument"=w183, "error in (no error)"=w186, "Python Object References In"=w189, "Session ID"=w192) -> ("error out"=w185:errorcluster, "Python Object References Out"=w188:T5, "Session ID out"=w191:T4)  [unwired: 5 in]
            n41 = call <vilib>:"Pack.vi"("Argument"=w182, "error in (no error)"=w185, "Python Object References In"=w188, "Session ID"=w191) -> ("error out"=w184:errorcluster, "Python Object References Out"=w187:T5, "Session ID out"=w190:T4)  [unwired: 5 in]
            n42 = call <vilib>:"Call.vi"("Function or Method Name"="AppendResultFile", "error in (no error)"=w184, "Python Object References In"=w187, "Session ID"=w190) -> ("error out"=w229:errorcluster, "Session ID out"=w220:T4)  [unwired: 5 in, 1 out]
            n43 = call <vilib>:"Close Session.vi"("error in (no error)"=w229, "Session ID"=w220) -> ()  [unwired: 9 in, 1 out]
            n44 = call <vilib>:"New Session.vi"("Path to Python Module (.py File)"=path "C:/Users/User/Documents/LabVIEW Data/2015 Projects/Combined/HPLCandAppendAmb.py") -> ("error out"=w211:errorcluster, "Session ID out"=w210:T4)  [unwired: 9 in]
            n45 = call <vilib>:"Pack.vi"("Argument"=w194, "error in (no error)"=w211, "Session ID"=w210) -> ("error out"=w196:errorcluster, "Python Object References Out"=w198:T5, "Session ID out"=w200:T4)  [unwired: 6 in]
            n46 = call <vilib>:"Pack.vi"("Argument"=w193, "error in (no error)"=w196, "Python Object References In"=w198, "Session ID"=w200) -> ("error out"=w195:errorcluster, "Python Object References Out"=w197:T5, "Session ID out"=w199:T4)  [unwired: 5 in]
            n47 = call <vilib>:"Call.vi"("Function or Method Name"="HPLC", "error in (no error)"=w195, "Python Object References In"=w197, "Session ID"=w199) -> ("error out"=w212:errorcluster, "Python Object References Out"=w203:T5, "Session ID out"=w204:T4)  [unwired: 5 in]
            n48 = call-poly <vilib>:"Unpack.vi"("error in (no error)"=w212, "Python Object References In"=w203, "Session ID"=w204) -> ("error out"=w213:errorcluster, "Value"=→"C BAcid 1":dbl, "Python Object References Out"=w208:T5, "Session ID out"=w207:T4)  [unwired: 5 in]
            n49 = call-poly <vilib>:"Unpack.vi"("error in (no error)"=w213, "Python Object References In"=w208, "Session ID"=w207) -> ("error out"=w214:errorcluster, "Value"=→"C EB 1":dbl, "Session ID out"=w209:T4)  [unwired: 5 in, 1 out]
            n50 = call <vilib>:"Close Session.vi"("error in (no error)"=w214, "Session ID"=w209) -> ()  [unwired: 9 in, 1 out]
            "Exp 9" <- TRUE
            "Temp 2" <- w217
            "Flow 2" <- w216
            "Conc 2" <- w215
          }
          frame 4 {
            n51 = flat-sequence {
              tunnel: w241 -> [w249]
              tunnel: w237 -> [w242]
              tunnel: w237 -> [_]
              tunnel: w237 -> [w293]
              tunnel: ["Temp 3"] -> w240
              tunnel: ["Flow 3"] -> w239
              tunnel: ["Conc 3"] -> w238
              tunnel: w235 -> [w289]
              tunnel: w234 -> [w288]
              frame #0 {
                # "make this include a write to record file step"
                n52 = call <vilib>:"New Session.vi"("Path to Python Module (.py File)"=path "C:/Users/User/Documents/LabVIEW Data/2015 Projects/Combined/HPLCandAppendAmb.py") -> ("error out"=w260:errorcluster, "Session ID out"=w259:T4)  [unwired: 9 in]
                n53 = call <vilib>:"Pack.vi"("Argument"=w249, "error in (no error)"=w260, "Session ID"=w259) -> ("error out"=w244:errorcluster, "Python Object References Out"=w246:T5, "Session ID out"=w248:T4)  [unwired: 6 in]
                n54 = call <vilib>:"Pack.vi"("Argument"=w242, "error in (no error)"=w244, "Python Object References In"=w246, "Session ID"=w248) -> ("error out"=w243:errorcluster, "Python Object References Out"=w245:T5, "Session ID out"=w247:T4)  [unwired: 5 in]
                n55 = call <vilib>:"Call.vi"("Function or Method Name"="HPLC", "error in (no error)"=w243, "Python Object References In"=w245, "Session ID"=w247) -> ("error out"=w261:errorcluster, "Python Object References Out"=w252:T5, "Session ID out"=w253:T4)  [unwired: 5 in]
                n56 = call-poly <vilib>:"Unpack.vi"("error in (no error)"=w261, "Python Object References In"=w252, "Session ID"=w253) -> ("error out"=w262:errorcluster, "Value"=→"C BAcid 2":dbl, "Python Object References Out"=w257:T5, "Session ID out"=w256:T4)  [unwired: 5 in]
                n57 = call-poly <vilib>:"Unpack.vi"("error in (no error)"=w262, "Python Object References In"=w257, "Session ID"=w256) -> ("error out"=w263:errorcluster, "Value"=→"C EB 2":dbl, "Session ID out"=w258:T4)  [unwired: 5 in, 1 out]
                n58 = call <vilib>:"Close Session.vi"("error in (no error)"=w263, "Session ID"=w258) -> ()  [unwired: 9 in, 1 out]
              }
              frame #1 {
              }
              frame #2 {
                n59 = call <vilib>:"New Session.vi"("Path to Python Module (.py File)"=path "C:/Users/User/Documents/LabVIEW Data/2015 Projects/Combined/WriteTFCDM.py") -> ("error out"=w281:errorcluster, "Session ID out"=w282:T4)  [unwired: 9 in]
                n60 = call <vilib>:"Pack.vi"("Argument"=w293, "error in (no error)"=w281, "Session ID"=w282) -> ("error out"=w280:errorcluster, "Python Object References Out"=w276:T5, "Session ID out"=w283:T4)  [unwired: 6 in]
                n61 = call <vilib>:"Pack.vi"("Argument"="Temp 3", "error in (no error)"=w280, "Python Object References In"=w276, "Session ID"=w283) -> ("error out"=w279:errorcluster, "Python Object References Out"=w275:T5, "Session ID out"=w273:T4)  [unwired: 5 in]
                n62 = call <vilib>:"Pack.vi"("Argument"="Flow 3", "error in (no error)"=w279, "Python Object References In"=w275, "Session ID"=w273) -> ("error out"=w278:errorcluster, "Python Object References Out"=w274:T5, "Session ID out"=w287:T4)  [unwired: 5 in]
                n63 = call <vilib>:"Pack.vi"("Argument"="Conc 3", "error in (no error)"=w278, "Python Object References In"=w274, "Session ID"=w287) -> ("error out"=w267:errorcluster, "Python Object References Out"=w269:T5, "Session ID out"=w272:T4)  [unwired: 5 in]
                n64 = call <vilib>:"Pack.vi"("Argument"=w289, "error in (no error)"=w267, "Python Object References In"=w269, "Session ID"=w272) -> ("error out"=w266:errorcluster, "Python Object References Out"=w268:T5, "Session ID out"=w271:T4)  [unwired: 5 in]
                n65 = call <vilib>:"Pack.vi"("Argument"=w288, "error in (no error)"=w266, "Python Object References In"=w268, "Session ID"=w271) -> ("error out"=w265:errorcluster, "Python Object References Out"=w264:T5, "Session ID out"=w270:T4)  [unwired: 5 in]
                n66 = call <vilib>:"Call.vi"("Function or Method Name"="AppendResultFile", "error in (no error)"=w265, "Python Object References In"=w264, "Session ID"=w270) -> ("error out"=w277:errorcluster, "Session ID out"=w286:T4)  [unwired: 5 in, 1 out]
                n67 = call <vilib>:"Close Session.vi"("error in (no error)"=w277, "Session ID"=w286) -> ()  [unwired: 9 in, 1 out]
                "Temp 3" <- "Temp 3"
                "Flow 3" <- "Flow 3"
                "Conc 3" <- "Conc 3"
              }
            }
            "Exp 3" <- TRUE
          }
          frame 5 {
            n68 = flat-sequence {
              tunnel: w301 -> [w309]
              tunnel: w297 -> [w302]
              tunnel: w297 -> [_]
              tunnel: w297 -> [w353]
              tunnel: ["Temp 4"] -> w300
              tunnel: ["Flow 4"] -> w299
              tunnel: ["Conc 4"] -> w298
              tunnel: w295 -> [w325]
              tunnel: w294 -> [w324]
              frame #0 {
                # "make this include a write to record file step"
                n69 = call <vilib>:"New Session.vi"("Path to Python Module (.py File)"=path "C:/Users/User/Documents/LabVIEW Data/2015 Projects/Combined/HPLCandAppendAmb.py") -> ("error out"=w320:errorcluster, "Session ID out"=w319:T4)  [unwired: 9 in]
                n70 = call <vilib>:"Pack.vi"("Argument"=w309, "error in (no error)"=w320, "Session ID"=w319) -> ("error out"=w304:errorcluster, "Python Object References Out"=w306:T5, "Session ID out"=w308:T4)  [unwired: 6 in]
                n71 = call <vilib>:"Pack.vi"("Argument"=w302, "error in (no error)"=w304, "Python Object References In"=w306, "Session ID"=w308) -> ("error out"=w303:errorcluster, "Python Object References Out"=w305:T5, "Session ID out"=w307:T4)  [unwired: 5 in]
                n72 = call <vilib>:"Call.vi"("Function or Method Name"="HPLC", "error in (no error)"=w303, "Python Object References In"=w305, "Session ID"=w307) -> ("error out"=w321:errorcluster, "Python Object References Out"=w312:T5, "Session ID out"=w313:T4)  [unwired: 5 in]
                n73 = call-poly <vilib>:"Unpack.vi"("error in (no error)"=w321, "Python Object References In"=w312, "Session ID"=w313) -> ("error out"=w322:errorcluster, "Value"=→"C BAcid 3":dbl, "Python Object References Out"=w317:T5, "Session ID out"=w316:T4)  [unwired: 5 in]
                n74 = call-poly <vilib>:"Unpack.vi"("error in (no error)"=w322, "Python Object References In"=w317, "Session ID"=w316) -> ("error out"=w323:errorcluster, "Value"=→"C EB 3":dbl, "Session ID out"=w318:T4)  [unwired: 5 in, 1 out]
                n75 = call <vilib>:"Close Session.vi"("error in (no error)"=w323, "Session ID"=w318) -> ()  [unwired: 9 in, 1 out]
              }
              frame #1 {
              }
              frame #2 {
                n76 = call <vilib>:"New Session.vi"("Path to Python Module (.py File)"=path "C:/Users/User/Documents/LabVIEW Data/2015 Projects/Combined/WriteTFCDM.py") -> ("error out"=w343:errorcluster, "Session ID out"=w344:T4)  [unwired: 9 in]
                n77 = call <vilib>:"Pack.vi"("Argument"=w353, "error in (no error)"=w343, "Session ID"=w344) -> ("error out"=w342:errorcluster, "Python Object References Out"=w338:T5, "Session ID out"=w345:T4)  [unwired: 6 in]
                n78 = call <vilib>:"Pack.vi"("Argument"="Temp 4", "error in (no error)"=w342, "Python Object References In"=w338, "Session ID"=w345) -> ("error out"=w341:errorcluster, "Python Object References Out"=w337:T5, "Session ID out"=w335:T4)  [unwired: 5 in]
                n79 = call <vilib>:"Pack.vi"("Argument"="Flow 4", "error in (no error)"=w341, "Python Object References In"=w337, "Session ID"=w335) -> ("error out"=w340:errorcluster, "Python Object References Out"=w336:T5, "Session ID out"=w349:T4)  [unwired: 5 in]
                n80 = call <vilib>:"Pack.vi"("Argument"="Conc 4", "error in (no error)"=w340, "Python Object References In"=w336, "Session ID"=w349) -> ("error out"=w328:errorcluster, "Python Object References Out"=w331:T5, "Session ID out"=w334:T4)  [unwired: 5 in]
                n81 = call <vilib>:"Pack.vi"("Argument"=w325, "error in (no error)"=w328, "Python Object References In"=w331, "Session ID"=w334) -> ("error out"=w327:errorcluster, "Python Object References Out"=w330:T5, "Session ID out"=w333:T4)  [unwired: 5 in]
                n82 = call <vilib>:"Pack.vi"("Argument"=w324, "error in (no error)"=w327, "Python Object References In"=w330, "Session ID"=w333) -> ("error out"=w326:errorcluster, "Python Object References Out"=w329:T5, "Session ID out"=w332:T4)  [unwired: 5 in]
                n83 = call <vilib>:"Call.vi"("Function or Method Name"="AppendResultFile", "error in (no error)"=w326, "Python Object References In"=w329, "Session ID"=w332) -> ("error out"=w339:errorcluster, "Session ID out"=w348:T4)  [unwired: 5 in, 1 out]
                n84 = call <vilib>:"Close Session.vi"("error in (no error)"=w339, "Session ID"=w348) -> ()  [unwired: 9 in, 1 out]
                "Temp 4" <- "Temp 4"
                "Flow 4" <- "Flow 4"
                "Conc 4" <- "Conc 4"
              }
            }
            "Exp 4" <- TRUE
          }
          frame 6 {
            n85 = flat-sequence {
              tunnel: w361 -> [w369]
              tunnel: w357 -> [w362]
              tunnel: w357 -> [w384]
              tunnel: w357 -> [w443]
              tunnel: ["Temp 5"] -> w360
              tunnel: ["Flow 5"] -> w359
              tunnel: ["Conc 5"] -> w358
              tunnel: w355 -> [w415]
              tunnel: w354 -> [w414]
              frame #0 {
                # "make this include a write to record file step"
                n86 = call <vilib>:"New Session.vi"("Path to Python Module (.py File)"=path "C:/Users/User/Documents/LabVIEW Data/2015 Projects/Combined/HPLCandAppendAmb.py") -> ("error out"=w380:errorcluster, "Session ID out"=w379:T4)  [unwired: 9 in]
                n87 = call <vilib>:"Pack.vi"("Argument"=w369, "error in (no error)"=w380, "Session ID"=w379) -> ("error out"=w366:errorcluster, "Python Object References Out"=w367:T5, "Session ID out"=w368:T4)  [unwired: 6 in]
                n88 = call <vilib>:"Pack.vi"("Argument"=w362, "error in (no error)"=w366, "Python Object References In"=w367, "Session ID"=w368) -> ("error out"=w365:errorcluster, "Python Object References Out"=w364:T5, "Session ID out"=w363:T4)  [unwired: 5 in]
                n89 = call <vilib>:"Call.vi"("Function or Method Name"="HPLC", "error in (no error)"=w365, "Python Object References In"=w364, "Session ID"=w363) -> ("error out"=w381:errorcluster, "Python Object References Out"=w372:T5, "Session ID out"=w373:T4)  [unwired: 5 in]
                n90 = call-poly <vilib>:"Unpack.vi"("error in (no error)"=w381, "Python Object References In"=w372, "Session ID"=w373) -> ("error out"=w382:errorcluster, "Value"=→"C BAcid 4":dbl, "Python Object References Out"=w377:T5, "Session ID out"=w376:T4)  [unwired: 5 in]
                n91 = call-poly <vilib>:"Unpack.vi"("error in (no error)"=w382, "Python Object References In"=w377, "Session ID"=w376) -> ("error out"=w383:errorcluster, "Value"=→"C EB 4":dbl, "Session ID out"=w378:T4)  [unwired: 5 in, 1 out]
                n92 = call <vilib>:"Close Session.vi"("error in (no error)"=w383, "Session ID"=w378) -> ()  [unwired: 9 in, 1 out]
              }
              frame #1 {
                n93 = call <vilib>:"New Session.vi"("Path to Python Module (.py File)"=path "C:/Users/User/Documents/LabVIEW Data/2015 Projects/Combined/Conor_PE_only_Amb_LabVIEW.py") -> ("error out"=w399:errorcluster, "Session ID out"=w396:T4)  [unwired: 9 in]
                n94 = call <vilib>:"Pack.vi"("Argument"=w384, "error in (no error)"=w399, "Session ID"=w396) -> ("error out"=w400:errorcluster, "Python Object References Out"=w398:T5, "Session ID out"=w397:T4)  [unwired: 6 in]
                n95 = call <vilib>:"Call.vi"("Function or Method Name"="PE_N_paramFive", "error in (no error)"=w400, "Python Object References In"=w398, "Session ID"=w397) -> ("error out"=w409:errorcluster, "Python Object References Out"=w405:T5, "Session ID out"=w401:T4)  [unwired: 5 in]
                n96 = call-poly <vilib>:"Unpack.vi"("error in (no error)"=w409, "Python Object References In"=w405, "Session ID"=w401) -> ("error out"=w410:errorcluster, "Value"=→"Param 1 4":dbl, "Python Object References Out"=w406:T5, "Session ID out"=w402:T4)  [unwired: 5 in]
                n97 = call-poly <vilib>:"Unpack.vi"("error in (no error)"=w410, "Python Object References In"=w406, "Session ID"=w402) -> ("error out"=w411:errorcluster, "Value"=→"Param 2 4":dbl, "Python Object References Out"=w407:T5, "Session ID out"=w403:T4)  [unwired: 5 in]
                n98 = call-poly <vilib>:"Unpack.vi"("error in (no error)"=w411, "Python Object References In"=w407, "Session ID"=w403) -> ("error out"=w412:errorcluster, "Value"=→"Param 3 4":dbl, "Python Object References Out"=w408:T5, "Session ID out"=w404:T4)  [unwired: 5 in]
                n99 = call-poly <vilib>:"Unpack.vi"("error in (no error)"=w412, "Python Object References In"=w408, "Session ID"=w404) -> ("error out"=w413:errorcluster, "Value"=→"Chi Sq 4":dbl, "Python Object References Out"=w395:T5, "Session ID out"=w394:T4)  [unwired: 5 in]
                n100 = call-poly <vilib>:"Unpack.vi"("error in (no error)"=w413, "Python Object References In"=w395, "Session ID"=w394) -> ("error out"=w390:errorcluster, "Value"=→"Chi Sq ref 4":dbl, "Session ID out"=w391:T4)  [unwired: 5 in, 1 out]
                n101 = call <vilib>:"Close Session.vi"("error in (no error)"=w390, "Session ID"=w391) -> ()  [unwired: 9 in, 1 out]
              }
              frame #2 {
                n102 = call <vilib>:"New Session.vi"("Path to Python Module (.py File)"=path "C:/Users/User/Documents/LabVIEW Data/2015 Projects/Combined/WriteTFCDM.py") -> ("error out"=w433:errorcluster, "Session ID out"=w434:T4)  [unwired: 9 in]
                n103 = call <vilib>:"Pack.vi"("Argument"=w443, "error in (no error)"=w433, "Session ID"=w434) -> ("error out"=w432:errorcluster, "Python Object References Out"=w428:T5, "Session ID out"=w435:T4)  [unwired: 6 in]
                n104 = call <vilib>:"Pack.vi"("Argument"="Temp 5", "error in (no error)"=w432, "Python Object References In"=w428, "Session ID"=w435) -> ("error out"=w431:errorcluster, "Python Object References Out"=w427:T5, "Session ID out"=w425:T4)  [unwired: 5 in]
                n105 = call <vilib>:"Pack.vi"("Argument"="Flow 5", "error in (no error)"=w431, "Python Object References In"=w427, "Session ID"=w425) -> ("error out"=w430:errorcluster, "Python Object References Out"=w426:T5, "Session ID out"=w439:T4)  [unwired: 5 in]
                n106 = call <vilib>:"Pack.vi"("Argument"="Conc 5", "error in (no error)"=w430, "Python Object References In"=w426, "Session ID"=w439) -> ("error out"=w418:errorcluster, "Python Object References Out"=w421:T5, "Session ID out"=w424:T4)  [unwired: 5 in]
                n107 = call <vilib>:"Pack.vi"("Argument"=w415, "error in (no error)"=w418, "Python Object References In"=w421, "Session ID"=w424) -> ("error out"=w417:errorcluster, "Python Object References Out"=w420:T5, "Session ID out"=w423:T4)  [unwired: 5 in]
                n108 = call <vilib>:"Pack.vi"("Argument"=w414, "error in (no error)"=w417, "Python Object References In"=w420, "Session ID"=w423) -> ("error out"=w416:errorcluster, "Python Object References Out"=w419:T5, "Session ID out"=w422:T4)  [unwired: 5 in]
                n109 = call <vilib>:"Call.vi"("Function or Method Name"="AppendResultFile", "error in (no error)"=w416, "Python Object References In"=w419, "Session ID"=w422) -> ("error out"=w429:errorcluster, "Session ID out"=w438:T4)  [unwired: 5 in, 1 out]
                n110 = call <vilib>:"Close Session.vi"("error in (no error)"=w429, "Session ID"=w438) -> ()  [unwired: 9 in, 1 out]
                "Temp 5" <- "Temp 5"
                "Flow 5" <- "Flow 5"
                "Conc 5" <- "Conc 5"
              }
            }
            "Exp 5" <- TRUE
          }
          frame 7 {
            n111 = flat-sequence {
              tunnel: w451 -> [w459]
              tunnel: w447 -> [w452]
              tunnel: w447 -> [w474]
              tunnel: w447 -> [w533]
              tunnel: ["Temp 6"] -> w450
              tunnel: ["Flow 6"] -> w449
              tunnel: ["Conc 6"] -> w448
              tunnel: w445 -> [w505]
              tunnel: w444 -> [w504]
              frame #0 {
                # "make this include a write to record file step"
                n112 = call <vilib>:"New Session.vi"("Path to Python Module (.py File)"=path "C:/Users/User/Documents/LabVIEW Data/2015 Projects/Combined/HPLCandAppendAmb.py") -> ("error out"=w470:errorcluster, "Session ID out"=w469:T4)  [unwired: 9 in]
                n113 = call <vilib>:"Pack.vi"("Argument"=w459, "error in (no error)"=w470, "Session ID"=w469) -> ("error out"=w456:errorcluster, "Python Object References Out"=w457:T5, "Session ID out"=w458:T4)  [unwired: 6 in]
                n114 = call <vilib>:"Pack.vi"("Argument"=w452, "error in (no error)"=w456, "Python Object References In"=w457, "Session ID"=w458) -> ("error out"=w453:errorcluster, "Python Object References Out"=w454:T5, "Session ID out"=w455:T4)  [unwired: 5 in]
                n115 = call <vilib>:"Call.vi"("Function or Method Name"="HPLC", "error in (no error)"=w453, "Python Object References In"=w454, "Session ID"=w455) -> ("error out"=w471:errorcluster, "Python Object References Out"=w462:T5, "Session ID out"=w463:T4)  [unwired: 5 in]
                n116 = call-poly <vilib>:"Unpack.vi"("error in (no error)"=w471, "Python Object References In"=w462, "Session ID"=w463) -> ("error out"=w472:errorcluster, "Value"=→"C BAcid 5":dbl, "Python Object References Out"=w467:T5, "Session ID out"=w466:T4)  [unwired: 5 in]
                n117 = call-poly <vilib>:"Unpack.vi"("error in (no error)"=w472, "Python Object References In"=w467, "Session ID"=w466) -> ("error out"=w473:errorcluster, "Value"=→"C EB 5":dbl, "Session ID out"=w468:T4)  [unwired: 5 in, 1 out]
                n118 = call <vilib>:"Close Session.vi"("error in (no error)"=w473, "Session ID"=w468) -> ()  [unwired: 9 in, 1 out]
              }
              frame #1 {
                n119 = call <vilib>:"New Session.vi"("Path to Python Module (.py File)"=path "C:/Users/User/Documents/LabVIEW Data/2015 Projects/Combined/Conor_PE_only_Amb_LabVIEW.py") -> ("error out"=w489:errorcluster, "Session ID out"=w486:T4)  [unwired: 9 in]
                n120 = call <vilib>:"Pack.vi"("Argument"=w474, "error in (no error)"=w489, "Session ID"=w486) -> ("error out"=w490:errorcluster, "Python Object References Out"=w488:T5, "Session ID out"=w487:T4)  [unwired: 6 in]
                n121 = call <vilib>:"Call.vi"("Function or Method Name"="PE_N_paramFive", "error in (no error)"=w490, "Python Object References In"=w488, "Session ID"=w487) -> ("error out"=w499:errorcluster, "Python Object References Out"=w495:T5, "Session ID out"=w491:T4)  [unwired: 5 in]
                n122 = call-poly <vilib>:"Unpack.vi"("error in (no error)"=w499, "Python Object References In"=w495, "Session ID"=w491) -> ("error out"=w500:errorcluster, "Value"=→"Param 1 5":dbl, "Python Object References Out"=w496:T5, "Session ID out"=w492:T4)  [unwired: 5 in]
                n123 = call-poly <vilib>:"Unpack.vi"("error in (no error)"=w500, "Python Object References In"=w496, "Session ID"=w492) -> ("error out"=w501:errorcluster, "Value"=→"Param 2 5":dbl, "Python Object References Out"=w497:T5, "Session ID out"=w493:T4)  [unwired: 5 in]
                n124 = call-poly <vilib>:"Unpack.vi"("error in (no error)"=w501, "Python Object References In"=w497, "Session ID"=w493) -> ("error out"=w502:errorcluster, "Value"=→"Param 3 5":dbl, "Python Object References Out"=w498:T5, "Session ID out"=w494:T4)  [unwired: 5 in]
                n125 = call-poly <vilib>:"Unpack.vi"("error in (no error)"=w502, "Python Object References In"=w498, "Session ID"=w494) -> ("error out"=w503:errorcluster, "Value"=→"Chi Sq 5":dbl, "Python Object References Out"=w485:T5, "Session ID out"=w484:T4)  [unwired: 5 in]
                n126 = call-poly <vilib>:"Unpack.vi"("error in (no error)"=w503, "Python Object References In"=w485, "Session ID"=w484) -> ("error out"=w480:errorcluster, "Value"=→"Chi Sq ref 5":dbl, "Session ID out"=w481:T4)  [unwired: 5 in, 1 out]
                n127 = call <vilib>:"Close Session.vi"("error in (no error)"=w480, "Session ID"=w481) -> ()  [unwired: 9 in, 1 out]
              }
              frame #2 {
                n128 = call <vilib>:"New Session.vi"("Path to Python Module (.py File)"=path "C:/Users/User/Documents/LabVIEW Data/2015 Projects/Combined/WriteTFCDM.py") -> ("error out"=w523:errorcluster, "Session ID out"=w524:T4)  [unwired: 9 in]
                n129 = call <vilib>:"Pack.vi"("Argument"=w533, "error in (no error)"=w523, "Session ID"=w524) -> ("error out"=w522:errorcluster, "Python Object References Out"=w518:T5, "Session ID out"=w525:T4)  [unwired: 6 in]
                n130 = call <vilib>:"Pack.vi"("Argument"="Temp 6", "error in (no error)"=w522, "Python Object References In"=w518, "Session ID"=w525) -> ("error out"=w521:errorcluster, "Python Object References Out"=w517:T5, "Session ID out"=w515:T4)  [unwired: 5 in]
                n131 = call <vilib>:"Pack.vi"("Argument"="Flow 6", "error in (no error)"=w521, "Python Object References In"=w517, "Session ID"=w515) -> ("error out"=w520:errorcluster, "Python Object References Out"=w516:T5, "Session ID out"=w529:T4)  [unwired: 5 in]
                n132 = call <vilib>:"Pack.vi"("Argument"="Conc 6", "error in (no error)"=w520, "Python Object References In"=w516, "Session ID"=w529) -> ("error out"=w508:errorcluster, "Python Object References Out"=w511:T5, "Session ID out"=w514:T4)  [unwired: 5 in]
                n133 = call <vilib>:"Pack.vi"("Argument"=w505, "error in (no error)"=w508, "Python Object References In"=w511, "Session ID"=w514) -> ("error out"=w507:errorcluster, "Python Object References Out"=w510:T5, "Session ID out"=w513:T4)  [unwired: 5 in]
                n134 = call <vilib>:"Pack.vi"("Argument"=w504, "error in (no error)"=w507, "Python Object References In"=w510, "Session ID"=w513) -> ("error out"=w506:errorcluster, "Python Object References Out"=w509:T5, "Session ID out"=w512:T4)  [unwired: 5 in]
                n135 = call <vilib>:"Call.vi"("Function or Method Name"="AppendResultFile", "error in (no error)"=w506, "Python Object References In"=w509, "Session ID"=w512) -> ("error out"=w519:errorcluster, "Session ID out"=w528:T4)  [unwired: 5 in, 1 out]
                n136 = call <vilib>:"Close Session.vi"("error in (no error)"=w519, "Session ID"=w528) -> ()  [unwired: 9 in, 1 out]
                "Temp 6" <- "Temp 6"
                "Flow 6" <- "Flow 6"
                "Conc 6" <- "Conc 6"
              }
            }
            "Exp 6" <- TRUE
          }
          frame 8 {
            n137 = flat-sequence {
              tunnel: w541 -> [w549]
              tunnel: w537 -> [w542]
              tunnel: w537 -> [w564]
              tunnel: w537 -> [w623]
              tunnel: ["Temp 7"] -> w540
              tunnel: ["Flow 7"] -> w539
              tunnel: ["Conc 7"] -> w538
              tunnel: w535 -> [w595]
              tunnel: w534 -> [w594]
              frame #0 {
                # "make this include a write to record file step"
                n138 = call <vilib>:"New Session.vi"("Path to Python Module (.py File)"=path "C:/Users/User/Documents/LabVIEW Data/2015 Projects/Combined/HPLCandAppendAmb.py") -> ("error out"=w560:errorcluster, "Session ID out"=w559:T4)  [unwired: 9 in]
                n139 = call <vilib>:"Pack.vi"("Argument"=w549, "error in (no error)"=w560, "Session ID"=w559) -> ("error out"=w544:errorcluster, "Python Object References Out"=w546:T5, "Session ID out"=w548:T4)  [unwired: 6 in]
                n140 = call <vilib>:"Pack.vi"("Argument"=w542, "error in (no error)"=w544, "Python Object References In"=w546, "Session ID"=w548) -> ("error out"=w543:errorcluster, "Python Object References Out"=w545:T5, "Session ID out"=w547:T4)  [unwired: 5 in]
                n141 = call <vilib>:"Call.vi"("Function or Method Name"="HPLC", "error in (no error)"=w543, "Python Object References In"=w545, "Session ID"=w547) -> ("error out"=w561:errorcluster, "Python Object References Out"=w552:T5, "Session ID out"=w553:T4)  [unwired: 5 in]
                n142 = call-poly <vilib>:"Unpack.vi"("error in (no error)"=w561, "Python Object References In"=w552, "Session ID"=w553) -> ("error out"=w562:errorcluster, "Value"=→"C BAcid 6":dbl, "Python Object References Out"=w557:T5, "Session ID out"=w556:T4)  [unwired: 5 in]
                n143 = call-poly <vilib>:"Unpack.vi"("error in (no error)"=w562, "Python Object References In"=w557, "Session ID"=w556) -> ("error out"=w563:errorcluster, "Value"=→"C EB 6":dbl, "Session ID out"=w558:T4)  [unwired: 5 in, 1 out]
                n144 = call <vilib>:"Close Session.vi"("error in (no error)"=w563, "Session ID"=w558) -> ()  [unwired: 9 in, 1 out]
              }
              frame #1 {
                n145 = call <vilib>:"New Session.vi"("Path to Python Module (.py File)"=path "C:/Users/User/Documents/LabVIEW Data/2015 Projects/Combined/Conor_PE_only_Amb_LabVIEW.py") -> ("error out"=w579:errorcluster, "Session ID out"=w576:T4)  [unwired: 9 in]
                n146 = call <vilib>:"Pack.vi"("Argument"=w564, "error in (no error)"=w579, "Session ID"=w576) -> ("error out"=w580:errorcluster, "Python Object References Out"=w578:T5, "Session ID out"=w577:T4)  [unwired: 6 in]
                n147 = call <vilib>:"Call.vi"("Function or Method Name"="PE_N_paramFive", "error in (no error)"=w580, "Python Object References In"=w578, "Session ID"=w577) -> ("error out"=w589:errorcluster, "Python Object References Out"=w585:T5, "Session ID out"=w581:T4)  [unwired: 5 in]
                n148 = call-poly <vilib>:"Unpack.vi"("error in (no error)"=w589, "Python Object References In"=w585, "Session ID"=w581) -> ("error out"=w590:errorcluster, "Value"=→"Param 1 6":dbl, "Python Object References Out"=w586:T5, "Session ID out"=w582:T4)  [unwired: 5 in]
                n149 = call-poly <vilib>:"Unpack.vi"("error in (no error)"=w590, "Python Object References In"=w586, "Session ID"=w582) -> ("error out"=w591:errorcluster, "Value"=→"Param 2 6":dbl, "Python Object References Out"=w587:T5, "Session ID out"=w583:T4)  [unwired: 5 in]
                n150 = call-poly <vilib>:"Unpack.vi"("error in (no error)"=w591, "Python Object References In"=w587, "Session ID"=w583) -> ("error out"=w592:errorcluster, "Value"=→"Param 3 6":dbl, "Python Object References Out"=w588:T5, "Session ID out"=w584:T4)  [unwired: 5 in]
                n151 = call-poly <vilib>:"Unpack.vi"("error in (no error)"=w592, "Python Object References In"=w588, "Session ID"=w584) -> ("error out"=w593:errorcluster, "Value"=→"Chi Sq 6":dbl, "Python Object References Out"=w575:T5, "Session ID out"=w574:T4)  [unwired: 5 in]
                n152 = call-poly <vilib>:"Unpack.vi"("error in (no error)"=w593, "Python Object References In"=w575, "Session ID"=w574) -> ("error out"=w570:errorcluster, "Value"=→"Chi Sq ref 6":dbl, "Session ID out"=w571:T4)  [unwired: 5 in, 1 out]
                n153 = call <vilib>:"Close Session.vi"("error in (no error)"=w570, "Session ID"=w571) -> ()  [unwired: 9 in, 1 out]
              }
              frame #2 {
                n154 = call <vilib>:"New Session.vi"("Path to Python Module (.py File)"=path "C:/Users/User/Documents/LabVIEW Data/2015 Projects/Combined/WriteTFCDM.py") -> ("error out"=w613:errorcluster, "Session ID out"=w614:T4)  [unwired: 9 in]
                n155 = call <vilib>:"Pack.vi"("Argument"=w623, "error in (no error)"=w613, "Session ID"=w614) -> ("error out"=w612:errorcluster, "Python Object References Out"=w608:T5, "Session ID out"=w615:T4)  [unwired: 6 in]
                n156 = call <vilib>:"Pack.vi"("Argument"="Temp 7", "error in (no error)"=w612, "Python Object References In"=w608, "Session ID"=w615) -> ("error out"=w611:errorcluster, "Python Object References Out"=w607:T5, "Session ID out"=w605:T4)  [unwired: 5 in]
                n157 = call <vilib>:"Pack.vi"("Argument"="Flow 7", "error in (no error)"=w611, "Python Object References In"=w607, "Session ID"=w605) -> ("error out"=w610:errorcluster, "Python Object References Out"=w606:T5, "Session ID out"=w619:T4)  [unwired: 5 in]
                n158 = call <vilib>:"Pack.vi"("Argument"="Conc 7", "error in (no error)"=w610, "Python Object References In"=w606, "Session ID"=w619) -> ("error out"=w598:errorcluster, "Python Object References Out"=w601:T5, "Session ID out"=w604:T4)  [unwired: 5 in]
                n159 = call <vilib>:"Pack.vi"("Argument"=w595, "error in (no error)"=w598, "Python Object References In"=w601, "Session ID"=w604) -> ("error out"=w597:errorcluster, "Python Object References Out"=w600:T5, "Session ID out"=w603:T4)  [unwired: 5 in]
                n160 = call <vilib>:"Pack.vi"("Argument"=w594, "error in (no error)"=w597, "Python Object References In"=w600, "Session ID"=w603) -> ("error out"=w596:errorcluster, "Python Object References Out"=w599:T5, "Session ID out"=w602:T4)  [unwired: 5 in]
                n161 = call <vilib>:"Call.vi"("Function or Method Name"="AppendResultFile", "error in (no error)"=w596, "Python Object References In"=w599, "Session ID"=w602) -> ("error out"=w609:errorcluster, "Session ID out"=w618:T4)  [unwired: 5 in, 1 out]
                n162 = call <vilib>:"Close Session.vi"("error in (no error)"=w609, "Session ID"=w618) -> ()  [unwired: 9 in, 1 out]
                "Temp 7" <- "Temp 7"
                "Flow 7" <- "Flow 7"
                "Conc 7" <- "Conc 7"
              }
            }
            "Exp 7" <- TRUE
          }
          frame 9 {
            n163 = flat-sequence {
              tunnel: w631 -> [w639]
              tunnel: w627 -> [w632]
              tunnel: w627 -> [w654]
              tunnel: w627 -> [w713]
              tunnel: ["Temp 8"] -> w630
              tunnel: ["Flow 8"] -> w629
              tunnel: ["Conc 8"] -> w628
              tunnel: w625 -> [w685]
              tunnel: w624 -> [w684]
              frame #0 {
                # "make this include a write to record file step"
                n164 = call <vilib>:"New Session.vi"("Path to Python Module (.py File)"=path "C:/Users/User/Documents/LabVIEW Data/2015 Projects/Combined/HPLCandAppendAmb.py") -> ("error out"=w650:errorcluster, "Session ID out"=w649:T4)  [unwired: 9 in]
                n165 = call <vilib>:"Pack.vi"("Argument"=w639, "error in (no error)"=w650, "Session ID"=w649) -> ("error out"=w636:errorcluster, "Python Object References Out"=w637:T5, "Session ID out"=w638:T4)  [unwired: 6 in]
                n166 = call <vilib>:"Pack.vi"("Argument"=w632, "error in (no error)"=w636, "Python Object References In"=w637, "Session ID"=w638) -> ("error out"=w635:errorcluster, "Python Object References Out"=w634:T5, "Session ID out"=w633:T4)  [unwired: 5 in]
                n167 = call <vilib>:"Call.vi"("Function or Method Name"="HPLC", "error in (no error)"=w635, "Python Object References In"=w634, "Session ID"=w633) -> ("error out"=w651:errorcluster, "Python Object References Out"=w642:T5, "Session ID out"=w643:T4)  [unwired: 5 in]
                n168 = call-poly <vilib>:"Unpack.vi"("error in (no error)"=w651, "Python Object References In"=w642, "Session ID"=w643) -> ("error out"=w652:errorcluster, "Value"=→"C BAcid 7":dbl, "Python Object References Out"=w647:T5, "Session ID out"=w646:T4)  [unwired: 5 in]
                n169 = call-poly <vilib>:"Unpack.vi"("error in (no error)"=w652, "Python Object References In"=w647, "Session ID"=w646) -> ("error out"=w653:errorcluster, "Value"=→"C EB 7":dbl, "Session ID out"=w648:T4)  [unwired: 5 in, 1 out]
                n170 = call <vilib>:"Close Session.vi"("error in (no error)"=w653, "Session ID"=w648) -> ()  [unwired: 9 in, 1 out]
              }
              frame #1 {
                n171 = call <vilib>:"New Session.vi"("Path to Python Module (.py File)"=path "C:/Users/User/Documents/LabVIEW Data/2015 Projects/Combined/Conor_PE_only_Amb_LabVIEW.py") -> ("error out"=w669:errorcluster, "Session ID out"=w666:T4)  [unwired: 9 in]
                n172 = call <vilib>:"Pack.vi"("Argument"=w654, "error in (no error)"=w669, "Session ID"=w666) -> ("error out"=w670:errorcluster, "Python Object References Out"=w668:T5, "Session ID out"=w667:T4)  [unwired: 6 in]
                n173 = call <vilib>:"Call.vi"("Function or Method Name"="PE_N_paramFive", "error in (no error)"=w670, "Python Object References In"=w668, "Session ID"=w667) -> ("error out"=w679:errorcluster, "Python Object References Out"=w675:T5, "Session ID out"=w671:T4)  [unwired: 5 in]
                n174 = call-poly <vilib>:"Unpack.vi"("error in (no error)"=w679, "Python Object References In"=w675, "Session ID"=w671) -> ("error out"=w680:errorcluster, "Value"=→"Param 1 7":dbl, "Python Object References Out"=w676:T5, "Session ID out"=w672:T4)  [unwired: 5 in]
                n175 = call-poly <vilib>:"Unpack.vi"("error in (no error)"=w680, "Python Object References In"=w676, "Session ID"=w672) -> ("error out"=w681:errorcluster, "Value"=→"Param 2 7":dbl, "Python Object References Out"=w677:T5, "Session ID out"=w673:T4)  [unwired: 5 in]
                n176 = call-poly <vilib>:"Unpack.vi"("error in (no error)"=w681, "Python Object References In"=w677, "Session ID"=w673) -> ("error out"=w682:errorcluster, "Value"=→"Param 3 7":dbl, "Python Object References Out"=w678:T5, "Session ID out"=w674:T4)  [unwired: 5 in]
                n177 = call-poly <vilib>:"Unpack.vi"("error in (no error)"=w682, "Python Object References In"=w678, "Session ID"=w674) -> ("error out"=w683:errorcluster, "Value"=→"Chi Sq 7":dbl, "Python Object References Out"=w665:T5, "Session ID out"=w664:T4)  [unwired: 5 in]
                n178 = call-poly <vilib>:"Unpack.vi"("error in (no error)"=w683, "Python Object References In"=w665, "Session ID"=w664) -> ("error out"=w660:errorcluster, "Value"=→"Chi Sq ref 7":dbl, "Session ID out"=w661:T4)  [unwired: 5 in, 1 out]
                n179 = call <vilib>:"Close Session.vi"("error in (no error)"=w660, "Session ID"=w661) -> ()  [unwired: 9 in, 1 out]
              }
              frame #2 {
                n180 = call <vilib>:"New Session.vi"("Path to Python Module (.py File)"=path "C:/Users/User/Documents/LabVIEW Data/2015 Projects/Combined/WriteTFCDM.py") -> ("error out"=w703:errorcluster, "Session ID out"=w704:T4)  [unwired: 9 in]
                n181 = call <vilib>:"Pack.vi"("Argument"=w713, "error in (no error)"=w703, "Session ID"=w704) -> ("error out"=w702:errorcluster, "Python Object References Out"=w698:T5, "Session ID out"=w705:T4)  [unwired: 6 in]
                n182 = call <vilib>:"Pack.vi"("Argument"="Temp 8", "error in (no error)"=w702, "Python Object References In"=w698, "Session ID"=w705) -> ("error out"=w701:errorcluster, "Python Object References Out"=w697:T5, "Session ID out"=w695:T4)  [unwired: 5 in]
                n183 = call <vilib>:"Pack.vi"("Argument"="Flow 8", "error in (no error)"=w701, "Python Object References In"=w697, "Session ID"=w695) -> ("error out"=w700:errorcluster, "Python Object References Out"=w696:T5, "Session ID out"=w709:T4)  [unwired: 5 in]
                n184 = call <vilib>:"Pack.vi"("Argument"="Conc 8", "error in (no error)"=w700, "Python Object References In"=w696, "Session ID"=w709) -> ("error out"=w688:errorcluster, "Python Object References Out"=w691:T5, "Session ID out"=w694:T4)  [unwired: 5 in]
                n185 = call <vilib>:"Pack.vi"("Argument"=w685, "error in (no error)"=w688, "Python Object References In"=w691, "Session ID"=w694) -> ("error out"=w687:errorcluster, "Python Object References Out"=w690:T5, "Session ID out"=w693:T4)  [unwired: 5 in]
                n186 = call <vilib>:"Pack.vi"("Argument"=w684, "error in (no error)"=w687, "Python Object References In"=w690, "Session ID"=w693) -> ("error out"=w686:errorcluster, "Python Object References Out"=w689:T5, "Session ID out"=w692:T4)  [unwired: 5 in]
                n187 = call <vilib>:"Call.vi"("Function or Method Name"="AppendResultFile", "error in (no error)"=w686, "Python Object References In"=w689, "Session ID"=w692) -> ("error out"=w699:errorcluster, "Session ID out"=w708:T4)  [unwired: 5 in, 1 out]
                n188 = call <vilib>:"Close Session.vi"("error in (no error)"=w699, "Session ID"=w708) -> ()  [unwired: 9 in, 1 out]
                "Temp 8" <- "Temp 8"
                "Flow 8" <- "Flow 8"
                "Conc 8" <- "Conc 8"
              }
            }
            "Exp 8" <- TRUE
          }
          frame 10 {
            n189 = flat-sequence {
              tunnel: w718 -> [w726]
              tunnel: w714 -> [w719]
              tunnel: w714 -> [w741]
              tunnel: w714 -> [_]
              frame #0 {
                # "make this include a write to record file step"
                n190 = call <vilib>:"New Session.vi"("Path to Python Module (.py File)"=path "C:/Users/User/Documents/LabVIEW Data/2015 Projects/Combined/HPLCandAppendAmb.py") -> ("error out"=w737:errorcluster, "Session ID out"=w736:T4)  [unwired: 9 in]
                n191 = call <vilib>:"Pack.vi"("Argument"=w726, "error in (no error)"=w737, "Session ID"=w736) -> ("error out"=w725:errorcluster, "Python Object References Out"=w724:T5, "Session ID out"=w723:T4)  [unwired: 6 in]
                n192 = call <vilib>:"Pack.vi"("Argument"=w719, "error in (no error)"=w725, "Python Object References In"=w724, "Session ID"=w723) -> ("error out"=w720:errorcluster, "Python Object References Out"=w721:T5, "Session ID out"=w722:T4)  [unwired: 5 in]
                n193 = call <vilib>:"Call.vi"("Function or Method Name"="HPLC", "error in (no error)"=w720, "Python Object References In"=w721, "Session ID"=w722) -> ("error out"=w738:errorcluster, "Python Object References Out"=w729:T5, "Session ID out"=w730:T4)  [unwired: 5 in]
                n194 = call-poly <vilib>:"Unpack.vi"("error in (no error)"=w738, "Python Object References In"=w729, "Session ID"=w730) -> ("error out"=w739:errorcluster, "Value"=→"C BAcid 8":dbl, "Python Object References Out"=w734:T5, "Session ID out"=w733:T4)  [unwired: 5 in]
                n195 = call-poly <vilib>:"Unpack.vi"("error in (no error)"=w739, "Python Object References In"=w734, "Session ID"=w733) -> ("error out"=w740:errorcluster, "Value"=→"C EB 8":dbl, "Session ID out"=w735:T4)  [unwired: 5 in, 1 out]
                n196 = call <vilib>:"Close Session.vi"("error in (no error)"=w740, "Session ID"=w735) -> ()  [unwired: 9 in, 1 out]
              }
              frame #1 {
                n197 = call <vilib>:"New Session.vi"("Path to Python Module (.py File)"=path "C:/Users/User/Documents/LabVIEW Data/2015 Projects/Combined/Conor_PE_only_Amb_LabVIEW.py") -> ("error out"=w756:errorcluster, "Session ID out"=w753:T4)  [unwired: 9 in]
                n198 = call <vilib>:"Pack.vi"("Argument"=w741, "error in (no error)"=w756, "Session ID"=w753) -> ("error out"=w757:errorcluster, "Python Object References Out"=w755:T5, "Session ID out"=w754:T4)  [unwired: 6 in]
                n199 = call <vilib>:"Call.vi"("Function or Method Name"="PE_N_paramFive", "error in (no error)"=w757, "Python Object References In"=w755, "Session ID"=w754) -> ("error out"=w766:errorcluster, "Python Object References Out"=w762:T5, "Session ID out"=w758:T4)  [unwired: 5 in]
                n200 = call-poly <vilib>:"Unpack.vi"("error in (no error)"=w766, "Python Object References In"=w762, "Session ID"=w758) -> ("error out"=w767:errorcluster, "Value"=→"Param 1 8":dbl, "Python Object References Out"=w763:T5, "Session ID out"=w759:T4)  [unwired: 5 in]
                n201 = call-poly <vilib>:"Unpack.vi"("error in (no error)"=w767, "Python Object References In"=w763, "Session ID"=w759) -> ("error out"=w768:errorcluster, "Value"=→"Param 2 8":dbl, "Python Object References Out"=w764:T5, "Session ID out"=w760:T4)  [unwired: 5 in]
                n202 = call-poly <vilib>:"Unpack.vi"("error in (no error)"=w768, "Python Object References In"=w764, "Session ID"=w760) -> ("error out"=w769:errorcluster, "Value"=→"Param 3 8":dbl, "Python Object References Out"=w765:T5, "Session ID out"=w761:T4)  [unwired: 5 in]
                n203 = call-poly <vilib>:"Unpack.vi"("error in (no error)"=w769, "Python Object References In"=w765, "Session ID"=w761) -> ("error out"=w770:errorcluster, "Value"=→"Chi Sq 8":dbl, "Python Object References Out"=w752:T5, "Session ID out"=w751:T4)  [unwired: 5 in]
                n204 = call-poly <vilib>:"Unpack.vi"("error in (no error)"=w770, "Python Object References In"=w752, "Session ID"=w751) -> ("error out"=w747:errorcluster, "Value"=→"Chi Sq ref 8":dbl, "Session ID out"=w748:T4)  [unwired: 5 in, 1 out]
                n205 = call <vilib>:"Close Session.vi"("error in (no error)"=w747, "Session ID"=w748) -> ()  [unwired: 9 in, 1 out]
              }
              frame #2 {
              }
            }
          }
        }
      }
      frame True {
        w771 = 0
      }
    }
    n206 = timed-loop {
      tunnel: w125 -> [w917]
      tunnel: w124 -> [w916]
      tunnel: [w865] -> w123
      tunnel: [w864] -> w122
      timing: w121 -> [_]
      timing-out: [_] -> w120
      tunnel: w119 -> [w851]
      tunnel: w118 -> [w855]
      tunnel: w117 -> [w854]
      tunnel: [w850] -> w116
      tunnel: [w849] -> w115
      tunnel: [w830] -> w114
      tunnel: w105 -> [w846]
      tunnel: w104 -> [w845]
      tunnel: w103 -> [w793]
      tunnel: w113 -> [w834]
      tunnel: w112 -> [w833]
      tunnel: w111 -> [w832]
      tunnel: w110 -> [w831]
      shift-right: [w794] -> _
      shift-left: _ -> [w825]
      tunnel: [w828] -> w109
      tunnel: [w827] -> w108
      tunnel: ["Stop everything"] -> w106
      tunnel: "Automated Experiments or Direct Control" -> [w795]
      tunnel: w92 -> [w788]
      tunnel: w91 -> [w787]
      tunnel: [w786] -> w90
      tunnel: [w785] -> w89
      i -> [w816]
      stop <- w823 stop-if-true
      w778 = 7.5 ("Safety Shut Down Pressure (barg)")
      w847 = 180
      # "Either pressures"
      # "in case out of range changes conc to within possible range"
      # "1st 4 flowrates\n5,6 temperatures\n7 pressure (1)\n8 gas (1)"
      # "temperature or syringe or gas or liquid pressure"
      # "We are graphing in barg"
      # "temperature or syringe"
      # "Empty Syringe has level of 50"
      n207 = node-c288() -> ()  [unwired: 1 in, 1 out]
      n208 = call-poly <vilib>:"DAQmx Read.vi"("task/channels in"=w788, "error in"=w787) -> ("task out"=w786:refnum<k21>, "data"=w781:dbl, "error out"=w785:errorcluster)  [unwired: 11 in]
      n209 = Multiply(x=5.1522, y=w781) -> (x*y=w784:dbl)
      n210 = Add(x=-2.6852, y=w784) -> (x+y=w779:dbl)
      "Liquid Inlet Pressure (bar g)" <- w779
      n211 = for {
        N: 4 -> [_]
        tunnel: w917 -> [w1187] mode=indexing
        tunnel: [w1185] -> w911 mode=indexing
        tunnel: [w1182] -> w906 mode=indexing
        tunnel: [w1181] -> w905 mode=indexing
        tunnel: [w1180] -> w904 mode=indexing
        tunnel: w916 -> [w1179] mode=indexing
        i -> [w1186]
        n212 = call "NCS_GetFlowRateIs.vi"("error in (no error)"=w1179, "dosingunit"=w1186, "device handle in"=w1187) -> ("error out"=w1183:errorcluster, "flowrate is"=w1185:dbl, "device handle out"=w1184:u32)
        n213 = call "NCS_GetSyringeLevelIs.vi"("error in (no error)"=w1183, "dosingunit"=w1186, "device handle in"=w1184) -> ("error out"=w1180:errorcluster, "syringe level is"=w1182:dbl, "device handle out"=w1181:u32)
      }
      n214 = Index Array(array=w906, index=0) -> (element=w820:dbl)
      "Syringe Level 1" <- w820
      n215 = Index Array(array=w906, index=3) -> (element=w817:dbl)
      "Syringe Level 4" <- w817
      n216 = Index Array(array=w906, index=1) -> (element=w819:dbl)
      "Syringe Level 2" <- w819
      n217 = Index Array(array=w906, index=2) -> (element=w818:dbl)
      "Syringe Level 3" <- w818
      n218 = case shown="True" "Shut down in empty?\nLeft off, right on" {
        tunnel: [FALSE w1088] -> w821
        tunnel: w820 -> [_ w1087]
        tunnel: w819 -> [_ w1086]
        tunnel: w818 -> [_ w1085]
        tunnel: w817 -> [_ w1084]
        frame False {
        }
        frame True {
          w1089 = 50
          n219 = Less Or Equal?(x=w1086, y=w1089) -> (x <= y?=w1095:bool)
          n220 = Less Or Equal?(x=w1087, y=w1089) -> (x <= y?=w1090:bool)
          n221 = Less Or Equal?(x=w1085, y=w1089) -> (x <= y?=w1093:bool)
          n222 = Less Or Equal?(x=w1084, y=w1089) -> (x <= y?=w1091:bool)
          n223 = Or(x=w1090, y=w1095) -> (x .or. y?=w1094:bool)
          n224 = Or(x=w1094, y=w1093) -> (x .or. y?=w1092:bool)
          n225 = Or(x=w1092, y=w1091) -> (x .or. y?=w1088:bool)
        }
      }
      n226 = Index Array(array=w911, index=0) -> (element=w805:dbl)
      "Flowrate 1 Low" <- w805
      n227 = Index Array(array=w911, index=3) -> (element=w807:dbl)
      "Flowrate 4 High" <- w807
      n228 = Index Array(array=w911, index=1) -> (element=w804:dbl)
      "Flowrate 2 Low" <- w804
      n229 = Index Array(array=w911, index=2) -> (element=w772:dbl)
      "Flowrate 3 High" <- w772
      n230 = case shown="False" "Clear" {
        tunnel: w825 -> [w1096 _]
        tunnel: [w1096 w1097] -> w824
        frame False {
        }
        frame True {
          n231 = Initialize Array(0, 1) -> (w1097:i32[])
        }
      }
      n232 = call-poly <vilib>:"DAQmx Read.vi"("task/channels in"=w834, "error in"=w833) -> ("task out"=w828:refnum<k21>, "data"=w839:dbl[], "error out"=w827:errorcluster)  [unwired: 11 in]
      n233 = Add(x=w805, y=w804) -> (x+y=w809:dbl)
      n234 = Add(x=w809, y=w772) -> (x+y=w808:dbl)
      n235 = Index Array(array=w839, index=0) -> (element=w837:dbl)
      n236 = Add(x=w808, y=w807) -> (x+y=w806:dbl)
      "Total Flowrate (uL/min)" <- w806
      n237 = Divide(x=w805, y=w806) -> (x/y=w799:dbl)
      n238 = Multiply(x=w837, y=w832) -> (x*y=w838:dbl)
      n239 = Multiply(x="Low Conc", y=w799) -> (x*y=w803:dbl)
      n240 = Divide(x=w772, y=w806) -> (x/y=w800:dbl)
      n241 = Add(x=w838, y=w831) -> (x+y=w835:dbl)
      n242 = Multiply(x="High Conc", y=w800) -> (x*y=w802:dbl)
      n243 = Add(x=w803, y=w802) -> (x+y=→"Feed Concentration (M)":dbl)
      n244 = In Range and Coerce(upper limit="High Conc", x=w793, lower limit="Low Conc") -> (coerced(x)=w790:dbl, In Range?=w792:bool)
      n245 = case shown="True" w792 {
        tunnel: [w920 w922] -> w791
        tunnel: w793 -> [_ w922]
        tunnel: w790 -> [w920 _]
        tunnel: [TRUE FALSE] -> w789
        frame False {
        }
        frame True {
        }
      }
      "Desired Conc Not Possible" <- w789
      n246 = Multiply(x=w835, y=0.0689476) -> (x*y=w780:dbl)
      "Gas Back Pressure (barg)" <- w780
      n247 = case shown="False" w795 {
        tunnel: [w1150 w1160] -> w902
        tunnel: w845 -> [w1146 _]
        tunnel: w791 -> [w1148 _]
        tunnel: "High Conc" -> [w1149 _]
        tunnel: "Low Conc" -> [w1147 _]
        frame False {
          # "h-s/h-l"
          # "s-l/h-l"
          # "high flow"
          # "low flow"
          # "2 syringes each"
          # "h-s"
          # "s-l"
          # "h-l"
          n248 = Subtract(x=w1149, y=w1147) -> (x-y=w1151:dbl)
          n249 = Subtract(x=w1148, y=w1147) -> (x-y=w1159:dbl)
          n250 = Subtract(x=w1149, y=w1148) -> (x-y=w1152:dbl)
          n251 = Divide(x=w1146, y=2) -> (x/y=w1157:dbl)
          n252 = Divide(x=w1152, y=w1151) -> (x/y=w1156:dbl)
          n253 = Divide(x=w1159, y=w1151) -> (x/y=w1155:dbl)
          n254 = Multiply(x=w1157, y=w1156) -> (x*y=w1154:dbl)
          n255 = Multiply(x=w1157, y=w1155) -> (x*y=w1153:dbl)
          n256 = Build Array(w1154, w1154, w1153, w1153) -> (w1150:dbl[])
        }
        frame True {
          n257 = Build Array("Set Flowrate 1", "Set Flowrate 2", "Set Flowrate 3", "Set Flowrate 4") -> (w1160:dbl[])
        }
      }
      n258 = Greater Or Equal?(x=w779, y=w778) -> (x >= y?=w777:bool)
      n259 = Build Array (concatenate)(w824, w780) -> (w794:dbl[])
      "Calculated Pressure" <- w794
      n260 = Greater Or Equal?(x=w780, y=w778) -> (x >= y?=w776:bool)
      n261 = Or(x=w777, y=w776) -> (x .or. y?=w775:bool)
      n262 = case shown="False" w795 {
        tunnel: [w1101 FALSE] -> w797
        tunnel: w816 -> [w1100 _]
        frame False {
          # "changes set points for each new exp"
          n263 = Equal?(x=w1100, y=0) -> (x = y?=w1101:bool)
        }
        frame True {
          # "at end of each exp"
          # "doesnt automatically change set point"
        }
      }
      n264 = Or(x=w797, y="Update Temperature Set Point") -> (x .or. y?=w857:bool)
      n265 = case shown="False" w857 {
        tunnel: w855 -> [w1105 w1113]
        tunnel: w854 -> [w1104 w1112]
        tunnel: [w1105 w1111] -> w853
        tunnel: [w1104 w1110] -> w852
        tunnel: w851 -> [_ w1109]
        tunnel: w795 -> [_ w1107]
        tunnel: w846 -> [_ w1106]
        frame False {
        }
        frame True {
          n266 = case shown="True" w1107 {
            tunnel: [w1114 "Set Point (oC)"] -> w1108
            tunnel: w1106 -> [w1114 _]
            frame False {
            }
            frame True {
            }
          }
          n267 = call "CN7500_Write Set Point Value.vi"("Target Set Point Value"=w1108, "error in (no error)"=w1112, "Controller Number"=w1109, "VISA In"=w1113) -> ("error out"=w1110:errorcluster, "VISA Out"=w1111:refnum<visa-resource-name>)  [unwired: 6 in]
        }
      }
      n268 = Or(x="Generate Flow", y=w797) -> (x .or. y?=w798:bool)
      n269 = case shown="True" w798 {
        tunnel: w905 -> [w1166 w1171]
        tunnel: w904 -> [w1165 w1170]
        tunnel: [w1165 w1169] -> w811
        tunnel: [w1166 w1168] -> w810
        tunnel: w902 -> [_ w1167]
        frame False {
        }
        frame True {
          n270 = for {
            N: 4 -> [_]
            tunnel: w1171 -> [w1178] mode=indexing
            tunnel: w1170 -> [w1177] mode=indexing
            tunnel: [w1176] -> w1169 mode=indexing
            tunnel: [w1175] -> w1168 mode=indexing
            tunnel: w1167 -> [w1173] mode=indexing
            i -> [w1174]
            n271 = call "NCS_GenerateFlow.vi"("error in (no error)"=w1177, "flowrate"=w1173, "dosingunit"=w1174, "device handle in"=w1178) -> ("error out"=w1176:errorcluster, "device handle out"=w1175:u32)
          }
        }
      }
      n272 = call "CN7500_Read Process Value.vi"("error in (no error)"=w852, "Controller Number"=w851, "VISA In"=w853) -> ("error out"=w850:errorcluster, "Set Point Value"=w841:dbl, "Process Value"=w842:dbl, "VISA Out"=w849:refnum<visa-resource-name>)  [unwired: 5 in]
      "Temp Set Point (oC)" <- w841
      "Actual Temp (oC)" <- w842
      n273 = Merge Signals(w842, w841) -> (→"Temperature":dynamicdata)
      n274 = Merge Signals(w805, w804, w772, w807, w842, w841, w780, w779) -> (w863:dynamicdata)
      n275 = Greater Or Equal?(x=w842, y=w847) -> (x >= y?=w844:bool)
      n276 = call "Write To Measurement File"("Signals"=w863) -> ()  [unwired: 16 in, 3 out]
      n277 = Index Array(array=w811, index=0) -> (element=w892:errorcluster)
      n278 = Index Array(array=w810, index=0) -> (element=w893:u32)
      n279 = Index Array(array=w811, index=3) -> (element=w882:errorcluster)
      n280 = Index Array(array=w811, index=2) -> (element=w884:errorcluster)
      n281 = Index Array(array=w811, index=1) -> (element=w886:errorcluster)
      n282 = Index Array(array=w810, index=3) -> (element=w883:u32)
      n283 = Index Array(array=w810, index=2) -> (element=w885:u32)
      n284 = Index Array(array=w810, index=1) -> (element=w887:u32)
      n285 = case shown="False" "Stop Dose 2" {
        tunnel: w887 -> [w1133 w1138]
        tunnel: w886 -> [w1132 w1137]
        tunnel: [w1133 w1136] -> w879
        tunnel: [w1132 w1135] -> w878
        frame False {
        }
        frame True {
          n286 = call "NCS_Stop.vi"("error in (no error)"=w1137, "dosingunit"=1, "device handle in"=w1138) -> ("error out"=w1135:errorcluster, "device handle out"=w1136:u32)
        }
      }
      n287 = case shown="False" "Stop Dose 1" {
        tunnel: w893 -> [w1140 w1145]
        tunnel: w892 -> [w1139 w1144]
        tunnel: [w1140 w1143] -> w881
        tunnel: [w1139 w1142] -> w880
        frame False {
        }
        frame True {
          n288 = call "NCS_Stop.vi"("error in (no error)"=w1144, "dosingunit"=0, "device handle in"=w1145) -> ("error out"=w1142:errorcluster, "device handle out"=w1143:u32)
        }
      }
      n289 = case shown="False" "Stop Dose 3" {
        tunnel: w885 -> [w1126 w1131]
        tunnel: w884 -> [w1125 w1130]
        tunnel: [w1126 w1129] -> w877
        tunnel: [w1125 w1128] -> w876
        frame False {
        }
        frame True {
          n290 = call "NCS_Stop.vi"("error in (no error)"=w1130, "dosingunit"=2, "device handle in"=w1131) -> ("error out"=w1128:errorcluster, "device handle out"=w1129:u32)
        }
      }
      n291 = case shown="False" "Stop Dose 4" {
        tunnel: w883 -> [w1119 w1124]
        tunnel: w882 -> [w1118 w1123]
        tunnel: [w1119 w1122] -> w875
        tunnel: [w1118 w1121] -> w874
        frame False {
        }
        frame True {
          n292 = call "NCS_Stop.vi"("error in (no error)"=w1123, "dosingunit"=3, "device handle in"=w1124) -> ("error out"=w1121:errorcluster, "device handle out"=w1122:u32)
        }
      }
      n293 = case shown="False" "Safety or Emergency Syringe Control" {
        tunnel: w881 -> [w930 w971]
        tunnel: w880 -> [w926 w970]
        tunnel: w879 -> [w929 w969]
        tunnel: w878 -> [w925 w968]
        tunnel: w877 -> [w928 w967]
        tunnel: w876 -> [w924 w966]
        tunnel: w875 -> [w927 w965]
        tunnel: w874 -> [w923 w964]
        tunnel: [w930 w941] -> w873
        tunnel: [w929 w940] -> w872
        tunnel: [w928 w939] -> w871
        tunnel: [w927 w938] -> w870
        tunnel: [w925 w937] -> w869
        tunnel: [w924 w936] -> w868
        tunnel: [w923 w935] -> w867
        tunnel: [w926 w931] -> w866
        frame False {
        }
        frame True {
          n294 = case shown="False" "Calibrate 2" {
            tunnel: w969 -> [w1070 w1075]
            tunnel: w968 -> [w1069 w1074]
            tunnel: [w1070 w1073] -> w958
            tunnel: [w1069 w1072] -> w957
            frame False {
            }
            frame True {
              n295 = call "NCS_Calibrate.vi"("error in (no error)"=w1074, "dosingunit"=1, "device handle in"=w1075) -> ("error out"=w1072:errorcluster, "device handle out"=w1073:u32)
            }
          }
          n296 = case shown="False" "Calibrate 3" {
            tunnel: w967 -> [w1063 w1068]
            tunnel: w966 -> [w1062 w1067]
            tunnel: [w1063 w1066] -> w956
            tunnel: [w1062 w1065] -> w955
            frame False {
            }
            frame True {
              n297 = call "NCS_Calibrate.vi"("error in (no error)"=w1067, "dosingunit"=2, "device handle in"=w1068) -> ("error out"=w1065:errorcluster, "device handle out"=w1066:u32)
            }
          }
          n298 = case shown="False" "Calibrate 1" {
            tunnel: w971 -> [w1077 w1082]
            tunnel: w970 -> [w1076 w1081]
            tunnel: [w1077 w1080] -> w960
            tunnel: [w1076 w1079] -> w959
            frame False {
            }
            frame True {
              n299 = call "NCS_Calibrate.vi"("error in (no error)"=w1081, "dosingunit"=0, "device handle in"=w1082) -> ("error out"=w1079:errorcluster, "device handle out"=w1080:u32)
            }
          }
          n300 = case shown="False" "Calibrate 4" {
            tunnel: w965 -> [w1056 w1061]
            tunnel: w964 -> [w1055 w1060]
            tunnel: [w1056 w1059] -> w954
            tunnel: [w1055 w1058] -> w953
            frame False {
            }
            frame True {
              n301 = call "NCS_Calibrate.vi"("error in (no error)"=w1060, "dosingunit"=3, "device handle in"=w1061) -> ("error out"=w1058:errorcluster, "device handle out"=w1059:u32)
            }
          }
          n302 = case shown="False" "Empty 2" {
            tunnel: w958 -> [w1036 w1040]
            tunnel: w957 -> [w1035 w1038]
            tunnel: [w1036 w1039] -> w944
            tunnel: [w1035 w1037] -> w945
            frame False {
            }
            frame True {
              w1042 = 1
              n303 = call "NCS_GetFlowRateMax.vi"("error in (no error)"=w1038, "dosingunit"=w1042, "device handle in"=w1040) -> ("error out"=w1043:errorcluster, "flow rate max"=w1041:dbl, "device handle out"=w1044:u32)
              n304 = call "NCS_EmptySyrige.vi"("error in (no error)"=w1043, "flowrate"=w1041, "dosingunit"=w1042, "device handle in"=w1044) -> ("error out"=w1037:errorcluster, "device handle out"=w1039:u32)
            }
          }
          n305 = case shown="False" "Empty 1" {
            tunnel: w960 -> [w1046 w1054]
            tunnel: w959 -> [w1045 w1051]
            tunnel: [w1046 w1052] -> w942
            tunnel: [w1045 w1049] -> w943
            frame False {
            }
            frame True {
              w1048 = 0
              n306 = call "NCS_GetFlowRateMax.vi"("error in (no error)"=w1051, "dosingunit"=w1048, "device handle in"=w1054) -> ("error out"=w1050:errorcluster, "flow rate max"=w1047:dbl, "device handle out"=w1053:u32)
              n307 = call "NCS_EmptySyrige.vi"("error in (no error)"=w1050, "flowrate"=w1047, "dosingunit"=w1048, "device handle in"=w1053) -> ("error out"=w1049:errorcluster, "device handle out"=w1052:u32)
            }
          }
          n308 = case shown="False" "Empty 3" {
            tunnel: w956 -> [w1026 w1027]
            tunnel: w955 -> [w1025 w1028]
            tunnel: [w1026 w1029] -> w946
            tunnel: [w1025 w1030] -> w947
            frame False {
            }
            frame True {
              w1032 = 2
              n309 = call "NCS_GetFlowRateMax.vi"("error in (no error)"=w1028, "dosingunit"=w1032, "device handle in"=w1027) -> ("error out"=w1033:errorcluster, "flow rate max"=w1031:dbl, "device handle out"=w1034:u32)
              n310 = call "NCS_EmptySyrige.vi"("error in (no error)"=w1033, "flowrate"=w1031, "dosingunit"=w1032, "device handle in"=w1034) -> ("error out"=w1030:errorcluster, "device handle out"=w1029:u32)
            }
          }
          n311 = case shown="False" "Empty 4" {
            tunnel: w954 -> [w1016 w1017]
            tunnel: w953 -> [w1015 w1018]
            tunnel: [w1016 w1020] -> w948
            tunnel: [w1015 w1019] -> w949
            frame False {
            }
            frame True {
              w1022 = 3
              n312 = call "NCS_GetFlowRateMax.vi"("error in (no error)"=w1018, "dosingunit"=w1022, "device handle in"=w1017) -> ("error out"=w1023:errorcluster, "flow rate max"=w1021:dbl, "device handle out"=w1024:u32)
              n313 = call "NCS_EmptySyrige.vi"("error in (no error)"=w1023, "flowrate"=w1021, "dosingunit"=w1022, "device handle in"=w1024) -> ("error out"=w1019:errorcluster, "device handle out"=w1020:u32)
            }
          }
          n314 = case shown="False" "Refill 2" {
            tunnel: w944 -> [w996 w1000]
            tunnel: w945 -> [w995 w998]
            tunnel: [w996 w999] -> w940
            tunnel: [w995 w997] -> w937
            frame False {
            }
            frame True {
              w1002 = 1
              n315 = call "NCS_GetFlowRateMax.vi"("error in (no error)"=w998, "dosingunit"=w1002, "device handle in"=w1000) -> ("error out"=w1003:errorcluster, "flow rate max"=w1001:dbl, "device handle out"=w1004:u32)
              n316 = call "NCS_RefillSyrige.vi"("error in (no error)"=w1003, "flowrate"=w1001, "dosingunit"=w1002, "device handle in"=w1004) -> ("error out"=w997:errorcluster, "device handle out"=w999:u32)
            }
          }
          n317 = case shown="False" "Refill 1" {
            tunnel: w942 -> [w1006 w1014]
            tunnel: w943 -> [w1005 w1011]
            tunnel: [w1006 w1012] -> w941
            tunnel: [w1005 w1009] -> w931
            frame False {
            }
            frame True {
              w1008 = 0
              n318 = call "NCS_GetFlowRateMax.vi"("error in (no error)"=w1011, "dosingunit"=w1008, "device handle in"=w1014) -> ("error out"=w1010:errorcluster, "flow rate max"=w1007:dbl, "device handle out"=w1013:u32)
              n319 = call "NCS_RefillSyrige.vi"("error in (no error)"=w1010, "flowrate"=w1007, "dosingunit"=w1008, "device handle in"=w1013) -> ("error out"=w1009:errorcluster, "device handle out"=w1012:u32)
            }
          }
          n320 = case shown="False" "Refill 3" {
            tunnel: w946 -> [w986 w987]
            tunnel: w947 -> [w985 w988]
            tunnel: [w986 w989] -> w939
            tunnel: [w985 w990] -> w936
            frame False {
            }
            frame True {
              w992 = 2
              n321 = call "NCS_GetFlowRateMax.vi"("error in (no error)"=w988, "dosingunit"=w992, "device handle in"=w987) -> ("error out"=w993:errorcluster, "flow rate max"=w991:dbl, "device handle out"=w994:u32)
              n322 = call "NCS_RefillSyrige.vi"("error in (no error)"=w993, "flowrate"=w991, "dosingunit"=w992, "device handle in"=w994) -> ("error out"=w990:errorcluster, "device handle out"=w989:u32)
            }
          }
          n323 = case shown="False" "Refill 4" {
            tunnel: w948 -> [w976 w977]
            tunnel: w949 -> [w975 w978]
            tunnel: [w976 w980] -> w938
            tunnel: [w975 w979] -> w935
            frame False {
            }
            frame True {
              w982 = 3
              n324 = call "NCS_GetFlowRateMax.vi"("error in (no error)"=w978, "dosingunit"=w982, "device handle in"=w977) -> ("error out"=w983:errorcluster, "flow rate max"=w981:dbl, "device handle out"=w984:u32)
              n325 = call "NCS_RefillSyrige.vi"("error in (no error)"=w983, "flowrate"=w981, "dosingunit"=w982, "device handle in"=w984) -> ("error out"=w979:errorcluster, "device handle out"=w980:u32)
            }
          }
        }
      }
      n326 = Or(x=w844, y=w821) -> (x .or. y?=w829:bool)
      n327 = Or(x=w829, y=w775) -> (x .or. y?=w830:bool)
      n328 = Multiply(x="Minutes between Exp", y=60) -> (x*y=w813:dbl)
      n329 = Divide(x=w813, y=5) -> (x/y=w814:dbl)
      n330 = Greater Or Equal?(x=w816, y=w814) -> (x >= y?=w859:bool)
      n331 = Or(x=w859, y=w830) -> (x .or. y?=w843:bool)
      n332 = Or(x="Skip Exp", y=w843) -> (x .or. y?=w860:bool)
      n333 = Or(x="Stop everything", y=w860) -> (x .or. y?=w823:bool)
      n334 = node-c288() -> ()  [unwired: 1 in, 1 out]
      n335 = Build Array(w873, w872, w871, w870) -> (w865:u32[])
      n336 = Build Array(w866, w869, w868, w867) -> (w864:errorcluster[])
      "loop ind" <- w816
      "Safety Shut Down Temp" <- w847
      "Safety Shut Down Pressure (barg)" <- w778
    }
    n337 = Or(x=w106, y=w114) -> (x .or. y?=w107:bool)
    n338 = node-c288(w120) -> ()  [unwired: 1 out]
  }
  n339 = call <vilib>:"DAQmx Stop Task.vi"("task/channels in"=w18, "error in"=w17) -> ("task out"=w20:refnum<k21>, "error out"=w19:errorcluster)  [unwired: 12 in]
  n340 = Index Array(array=w47, index=0) -> (element=w49:u32)
  n341 = Index Array(array=w46, index=0) -> (element=w48:errorcluster)
  n342 = call <vilib>:"DAQmx Stop Task.vi"("task/channels in"=w7, "error in"=w5) -> ("task out"=w6:refnum<k21>, "error out"=w8:errorcluster)  [unwired: 12 in]
  n343 = call <vilib>:"DAQmx Clear Task.vi"("task in"=w20, "error in"=w19) -> ()  [unwired: 13 in, 1 out]
  n344 = call <vilib>:"DAQmx Clear Task.vi"("task in"=w6, "error in"=w8) -> ()  [unwired: 13 in, 1 out]
  n345 = call "NCS_CloseDevice.vi"("error in (no error)"=w48, "device handle"=w49) -> ()  [unwired: 1 out]
  n346 = call "CN7500_Write Set Point Value.vi"("Target Set Point Value"=25, "error in (no error)"=w35, "Controller Number"=w38, "VISA In"=w34) -> ("error out"=w40:errorcluster, "VISA Out"=w41:refnum<visa-resource-name>)  [unwired: 6 in]
  n347 = call "CN7500_Close.vi"("error in (no error)"=w40, "VISA resource name"=w41) -> ()  [unwired: 9 in, 1 out]
